vi "ACT_Loop.vi"() -> ()   [LabVIEW 2023, in "2024 AdvSwerve_ACT.lvlib"]
uses:
  2024 AdvSwerve_ACT.lvlib
  Cluster_CMD_ACT_Data.ctl
  ENUM_CMD_Mode Select.ctl
  Shared Code/TypeDefs/Cluster_CMD_Direction Data.ctl
  Shared Code/TypeDefs/Cluster_Module Velocity-Direction-Rotations.ctl
  Shared Code/TypeDefs/Level_Velocity plus-minus 1.ctl
  Shared Code/TypeDefs/Dial_Compase heading unit circle CCW positive.ctl
  Shared Code/TypeDefs/Cluster_X-Y.ctl
  Cluster_HW Output Values.ctl
  Shared Code/TypeDefs/Cluster_Swerve 4 Steer and Velocity.ctl
  Cluster_System Output Data.ctl
  Cluster_System Config_Values.ctl
  Shared Code/TypeDefs/Cluster_SW PID Config.ctl
  Shared Code/TypeDefs/Cluster_PID Gains.ctl
  Shared Code/TypeDefs/Cluster_High-Low.ctl
  Type Defs/Cluster_Length and Width.ctl
  Shared Code/TypeDefs/Cluster_Config_Swerve_Drive Param.ctl
  Shared Code/TypeDefs/Cluster_Config_Swerve_Steer Parm.ctl
  Cluster_Config Specific HW Values.ctl
  Cluster_Config Specific Data.ctl
  Shared Code/TypeDefs/ENUM_Module Position.ctl
  Cluster_Config Steer HW Values.ctl
  Shared Code/TypeDefs/Cluster_SparkMax Config_Motor Output.ctl
  <vilib>/Rock Robotics/WPI/ThirdParty/REV Robotics/REVLib/Typedef/Spark MAX Idle Mode.ctl
  Shared Code/TypeDefs/Cluster_Spark MAX Config_SLOT PID Config.ctl
  Shared Code/TypeDefs/Cluster_SparkMax Config_Smart Motion Parameters.ctl
  Cluster_Config Drive HW Values.ctl
  ENUM_ACT_State.ctl
  <vilib>/Rock Robotics/WPI/ThirdParty/Phoenix-LabVIEW/Motor Controller/Controls/CTRE_Phoenix_MotorControl_ControlMode.ctl
  <vilib>/Rock Robotics/WPI/MotorControl/WPI_MotorControlDeviceRef.ctl
  <vilib>/Rock Robotics/WPI/MotorControl/WPI_MotorControlType.ctl
  <vilib>/Rock Robotics/SystemInterfaces/DIO/FPGA_DIOPWMChannel.ctl
  <vilib>/Rock Robotics/WPI/PWM/WPI_PWMDeadband.ctl
  <vilib>/Rock Robotics/SystemInterfaces/DIO/FPGA_DIOChannel.ctl
  <vilib>/Rock Robotics/WPI/ThirdParty/Phoenix-LabVIEW/CANCoder/Controls/CTRE_Phoenix_CANcoder_DeviceRef.ctl
  ENUM_ACT_Action.ctl
  4f1f8321-3dc8-4b28-8619-20673fc77ec2.vi
  cbff3d61-3b62-444e-9844-795ae03579cd.vi
  089052c0-d540-4a78-a5cc-aeb70dbb496b.vi
  6201c2b1-dcd8-4430-86f1-9b4ee56c7753.vi
  b5508d6c-c1cc-4273-80c5-2077d34e1483.vi
  5f725c2a-0ce1-4524-8967-e83b15fdce90.vi
  bd5da564-2e8e-4505-86fc-30918feadaa2.vi
  8beda75f-c59a-4462-acc7-7c37ceab3777.vi
  47a9b741-f4a3-48b6-ae85-4ba2e502368e.vi
  e2e8a241-7810-4d95-85fd-17f3a55957a8.vi
  80d407e5-f582-430c-986f-ecd413765478.vi
  573e44c0-11f4-4bd9-ad56-904ec25dba75.vi
  e7494af9-f670-4352-9dfa-ae6ce50709ea.vi
  <vilib>/Utility/error.llb/Trim Whitespace.vi
  5f725c2a-0ce1-4524-8967-e83b15fdce90.vi/958b2683-dd4b-41b7-8ed1-41c95f63cef0.vi
  5f725c2a-0ce1-4524-8967-e83b15fdce90.vi/95f5fa9b-6175-4b34-88ee-cece92c38279.vi
  bd5da564-2e8e-4505-86fc-30918feadaa2.vi/958b2683-dd4b-41b7-8ed1-41c95f63cef0.vi
  bd5da564-2e8e-4505-86fc-30918feadaa2.vi/95f5fa9b-6175-4b34-88ee-cece92c38279.vi
  8beda75f-c59a-4462-acc7-7c37ceab3777.vi/958b2683-dd4b-41b7-8ed1-41c95f63cef0.vi
  8beda75f-c59a-4462-acc7-7c37ceab3777.vi/95f5fa9b-6175-4b34-88ee-cece92c38279.vi
  47a9b741-f4a3-48b6-ae85-4ba2e502368e.vi/958b2683-dd4b-41b7-8ed1-41c95f63cef0.vi
  47a9b741-f4a3-48b6-ae85-4ba2e502368e.vi/95f5fa9b-6175-4b34-88ee-cece92c38279.vi
  e2e8a241-7810-4d95-85fd-17f3a55957a8.vi/958b2683-dd4b-41b7-8ed1-41c95f63cef0.vi
  e2e8a241-7810-4d95-85fd-17f3a55957a8.vi/95f5fa9b-6175-4b34-88ee-cece92c38279.vi
  80d407e5-f582-430c-986f-ecd413765478.vi/958b2683-dd4b-41b7-8ed1-41c95f63cef0.vi
  80d407e5-f582-430c-986f-ecd413765478.vi/95f5fa9b-6175-4b34-88ee-cece92c38279.vi
  573e44c0-11f4-4bd9-ad56-904ec25dba75.vi/958b2683-dd4b-41b7-8ed1-41c95f63cef0.vi
  573e44c0-11f4-4bd9-ad56-904ec25dba75.vi/95f5fa9b-6175-4b34-88ee-cece92c38279.vi
  e7494af9-f670-4352-9dfa-ae6ce50709ea.vi/958b2683-dd4b-41b7-8ed1-41c95f63cef0.vi
  e7494af9-f670-4352-9dfa-ae6ce50709ea.vi/95f5fa9b-6175-4b34-88ee-cece92c38279.vi
  <vilib>/Utility/error.llb/Trim Whitespace One-Sided.vi
  5f725c2a-0ce1-4524-8967-e83b15fdce90.vi/95f5fa9b-6175-4b34-88ee-cece92c38279.vi/1c6bd52c-bbca-4d4a-a290-93ea2703fded.vi
  5f725c2a-0ce1-4524-8967-e83b15fdce90.vi/95f5fa9b-6175-4b34-88ee-cece92c38279.vi/47c2b0d5-b5fa-444e-9535-611565d375db.vi
  bd5da564-2e8e-4505-86fc-30918feadaa2.vi/95f5fa9b-6175-4b34-88ee-cece92c38279.vi/1c6bd52c-bbca-4d4a-a290-93ea2703fded.vi
  bd5da564-2e8e-4505-86fc-30918feadaa2.vi/95f5fa9b-6175-4b34-88ee-cece92c38279.vi/47c2b0d5-b5fa-444e-9535-611565d375db.vi
  8beda75f-c59a-4462-acc7-7c37ceab3777.vi/95f5fa9b-6175-4b34-88ee-cece92c38279.vi/1c6bd52c-bbca-4d4a-a290-93ea2703fded.vi
  8beda75f-c59a-4462-acc7-7c37ceab3777.vi/95f5fa9b-6175-4b34-88ee-cece92c38279.vi/47c2b0d5-b5fa-444e-9535-611565d375db.vi
  47a9b741-f4a3-48b6-ae85-4ba2e502368e.vi/95f5fa9b-6175-4b34-88ee-cece92c38279.vi/1c6bd52c-bbca-4d4a-a290-93ea2703fded.vi
  47a9b741-f4a3-48b6-ae85-4ba2e502368e.vi/95f5fa9b-6175-4b34-88ee-cece92c38279.vi/47c2b0d5-b5fa-444e-9535-611565d375db.vi
  e2e8a241-7810-4d95-85fd-17f3a55957a8.vi/95f5fa9b-6175-4b34-88ee-cece92c38279.vi/1c6bd52c-bbca-4d4a-a290-93ea2703fded.vi
  e2e8a241-7810-4d95-85fd-17f3a55957a8.vi/95f5fa9b-6175-4b34-88ee-cece92c38279.vi/47c2b0d5-b5fa-444e-9535-611565d375db.vi
  80d407e5-f582-430c-986f-ecd413765478.vi/95f5fa9b-6175-4b34-88ee-cece92c38279.vi/1c6bd52c-bbca-4d4a-a290-93ea2703fded.vi
  80d407e5-f582-430c-986f-ecd413765478.vi/95f5fa9b-6175-4b34-88ee-cece92c38279.vi/47c2b0d5-b5fa-444e-9535-611565d375db.vi
  573e44c0-11f4-4bd9-ad56-904ec25dba75.vi/95f5fa9b-6175-4b34-88ee-cece92c38279.vi/1c6bd52c-bbca-4d4a-a290-93ea2703fded.vi
  573e44c0-11f4-4bd9-ad56-904ec25dba75.vi/95f5fa9b-6175-4b34-88ee-cece92c38279.vi/47c2b0d5-b5fa-444e-9535-611565d375db.vi
  e7494af9-f670-4352-9dfa-ae6ce50709ea.vi/95f5fa9b-6175-4b34-88ee-cece92c38279.vi/1c6bd52c-bbca-4d4a-a290-93ea2703fded.vi
  e7494af9-f670-4352-9dfa-ae6ce50709ea.vi/95f5fa9b-6175-4b34-88ee-cece92c38279.vi/47c2b0d5-b5fa-444e-9535-611565d375db.vi
  RoboRIO Utilities/Global_STOP.vi
  Global_CMD_ACT_Data In.vi
  PigeonIMU/Global_SEN_Data Out.vi
  Global_ACT_Data Out.vi
  <vilib>/Utility/Data Type/Get Type Information.vi
  Shared Code/Utility/RWA/RWA/File/RWA_PC FIle Read String.vi
  Shared Code/Utility/RWA/RWA/Read Write Anything/RWA_File String.vi
  Shared Code/Utility/RWA/RWA/File/RWA_PC File Write String.vi
  <vilib>/Comparison/Equal/Equal Functor/Equal Functor.lvclass
  PigeonIMU/PigeonIMU_SEN_ts.lvlib
panel:
  in  "Set Steer Start Values":bool
  in  "Config Drive":T1={"Drive HW Ver"=0, "SparkMax Output"={"Motor Invert"=FALSE, "Ramp Rate OL (S)"=1.0, "Dead Band"=0.0, "Idle Mode"=enum."Coast"}, "Slot 0 CL"={"Gains"={"P"=0.1, "I"=0.0, "D"=0.0, "F"=0.0}, "I Zone"=0.0, "Peak Out -1 0 1"={"High"=0.0, "Low"=0.0}, "Max I Accu"=0.0}, "Slot 0 SM"={"Max Velocity"=0.0, "Max Acceleration"=0.0, "Allowed CL Error"=0.0, "Min Velocity Output"=0.0}} {"Slot 0 CL"."Gains"."F" format="%#.8f"; "Slot 0 CL"."Gains"."D" format="%#.8f"; "Slot 0 CL"."Gains"."I" format="%#.8f"; "Slot 0 CL"."Gains"."P" format="%#.8f"; "Slot 0 CL"."Peak Out -1 0 1"."Low" format="%#.8f"; "Slot 0 CL"."Peak Out -1 0 1"."High" format="%#.8f"}
  in  "Config Steer":T8={"Steer HW Ver"=0, "SparkMax Output"={"Motor Invert"=FALSE, "Ramp Rate OL (S)"=1.0, "Dead Band"=0.0, "Idle Mode"=enum."Coast"}, "Slot 0 CL"={"Gains"={"P"=1.0, "I"=0.01, "D"=0.0, "F"=0.0}, "I Zone"=10000.0, "Peak Out -1 0 1"={"High"=1.0, "Low"=-1.0}, "Max I Accu"=-1000.0}, "Slot 0 SM"={"Max Velocity"=5000.0, "Max Acceleration"=5000.0, "Allowed CL Error"=0.0, "Min Velocity Output"=0.0}} {"Slot 0 CL"."Gains"."F" format="%#.8f"; "Slot 0 CL"."Gains"."D" format="%#.8f"; "Slot 0 CL"."Gains"."I" format="%#.8f"; "Slot 0 CL"."Gains"."P" format="%#.8f"; "Slot 0 CL"."Peak Out -1 0 1"."Low" format="%#.8f"; "Slot 0 CL"."Peak Out -1 0 1"."High" format="%#.8f"}
  in  "Config Specific":T9={"Specific HW Ver"=0, "Specific Data"=[{"Motor Pos"=enum."Left-Front", "CAN Bus"="", "NEO Drive ID"=0, "NEO-Cancoder SteerID"=0, "Encoder Start Value"=0.0}, {"Motor Pos"=enum."Right-Front", "CAN Bus"="", "NEO Drive ID"=0, "NEO-Cancoder SteerID"=0, "Encoder Start Value"=0.0}, {"Motor Pos"=enum."Right-Back", "CAN Bus"="", "NEO Drive ID"=0, "NEO-Cancoder SteerID"=0, "Encoder Start Value"=0.0}, {"Motor Pos"=enum."Left-Back", "CAN Bus"="", "NEO Drive ID"=0, "NEO-Cancoder SteerID"=0, "Encoder Start Value"=0.0}]}
  in  "CMD Override":T12(tab)
  in  "Overide CMD":T13 {"Target Auto Angle" scale format="%.3f"; "Direction"."Rotate(Yaw) CCW 1 CW -1" scale=1.0..-1.0; "Direction"."Traverse"."Angle" scale format="%.3f"; "Direction"."Traverse"."Velocity" scale=-1.0..1.0 scale format="%.1f"}
  in  "Overide 1":bool caption="Overide"
  in  "Target Auto Angle":T18 scale format="%.3f"
  in  "Overide 2":bool caption="Overide"
  out "Current Time":timestamp
  in  "Config System":T20={"System Ver"=0, "Auto Angle PID"={"Gains"={"P"=0.1, "I"=0.0, "D"=0.0, "F"=0.0}, "Error Allowed"={"High"=0.0, "Low"=0.0}, "I Zone"={"High"=0.0, "Low"=0.0}, "Peak Out 0-1"={"High"=0.0, "Low"=0.0}, "Max I Accu"={"High"=0.0, "Low"=0.0}}, "Frame"={"Length"=33.0, "Width"=18.0}, "Drive Data"={"CPR"=14.0, "RevMotor/Wheel"=6.67, "Wheel Diameter (in)"=4.0}, "Speed Full Scale"=5000.0, "Steer Data"={"CPR"=1024.0}} {"Auto Angle PID"."Max I Accu"."Low" format="%#.8f"; "Auto Angle PID"."Max I Accu"."High" format="%#.8f"; "Auto Angle PID"."Gains"."F" format="%#.8f"; "Auto Angle PID"."Gains"."D" format="%#.8f"; "Auto Angle PID"."Gains"."I" format="%#.8f"; "Auto Angle PID"."Gains"."P" format="%#.8f"; "Auto Angle PID"."Error Allowed"."Low" format="%#.8f"; "Auto Angle PID"."Error Allowed"."High" format="%#.8f"; "Auto Angle PID"."I Zone"."Low" format="%#.8f"; "Auto Angle PID"."I Zone"."High" format="%#.8f"; "Auto Angle PID"."Peak Out 0-1"."Low" format="%#.8f"; "Auto Angle PID"."Peak Out 0-1"."High" format="%#.8f"}
  out "System Config":T25
  out "Sensor Read time":dbl format="%.3g"
  out "HW Output":T26 {"Swerve Read"."Back Right"."Angle" scale format="%.3f"; "Swerve Read"."Back Right"."Velocity" scale=-1.0..1.0 scale format="%.1f"; "Swerve Read"."Back Left"."Angle" scale format="%.3f"; "Swerve Read"."Back Left"."Velocity" scale=-1.0..1.0 scale format="%.1f"; "Swerve Read"."Front Left"."Angle" scale format="%.3f"; "Swerve Read"."Front Left"."Velocity" scale=-1.0..1.0 scale format="%.1f"; "Swerve Read"."Front Right"."Angle" scale format="%.3f"; "Swerve Read"."Front Right"."Velocity" scale=-1.0..1.0 scale format="%.1f"; "Pigeon Heading" scale format="%.3f"}
  in  "Read Saved Config":bool
  in  "Update Config":bool
  out "CMD":T13 {"Target Auto Angle" scale format="%.3f"; "Direction"."Rotate(Yaw) CCW 1 CW -1" scale=1.0..-1.0; "Direction"."Traverse"."Angle" scale format="%.3f"; "Direction"."Traverse"."Velocity" scale=-1.0..1.0 scale format="%.1f"}
  out "Cycle Time (S)":dbl format="%.3g"
  # "Teleop\nAuto"
  # "STOP"
  # "\"Front\" of Robot"
  # "Index 1"
  # "Index 0"
  # "Index 3"
  # "Index 2"
  # "Right Hand Rule"
  # "X"
  # "+CCW"
  # "Y"
  # "(0,0)"
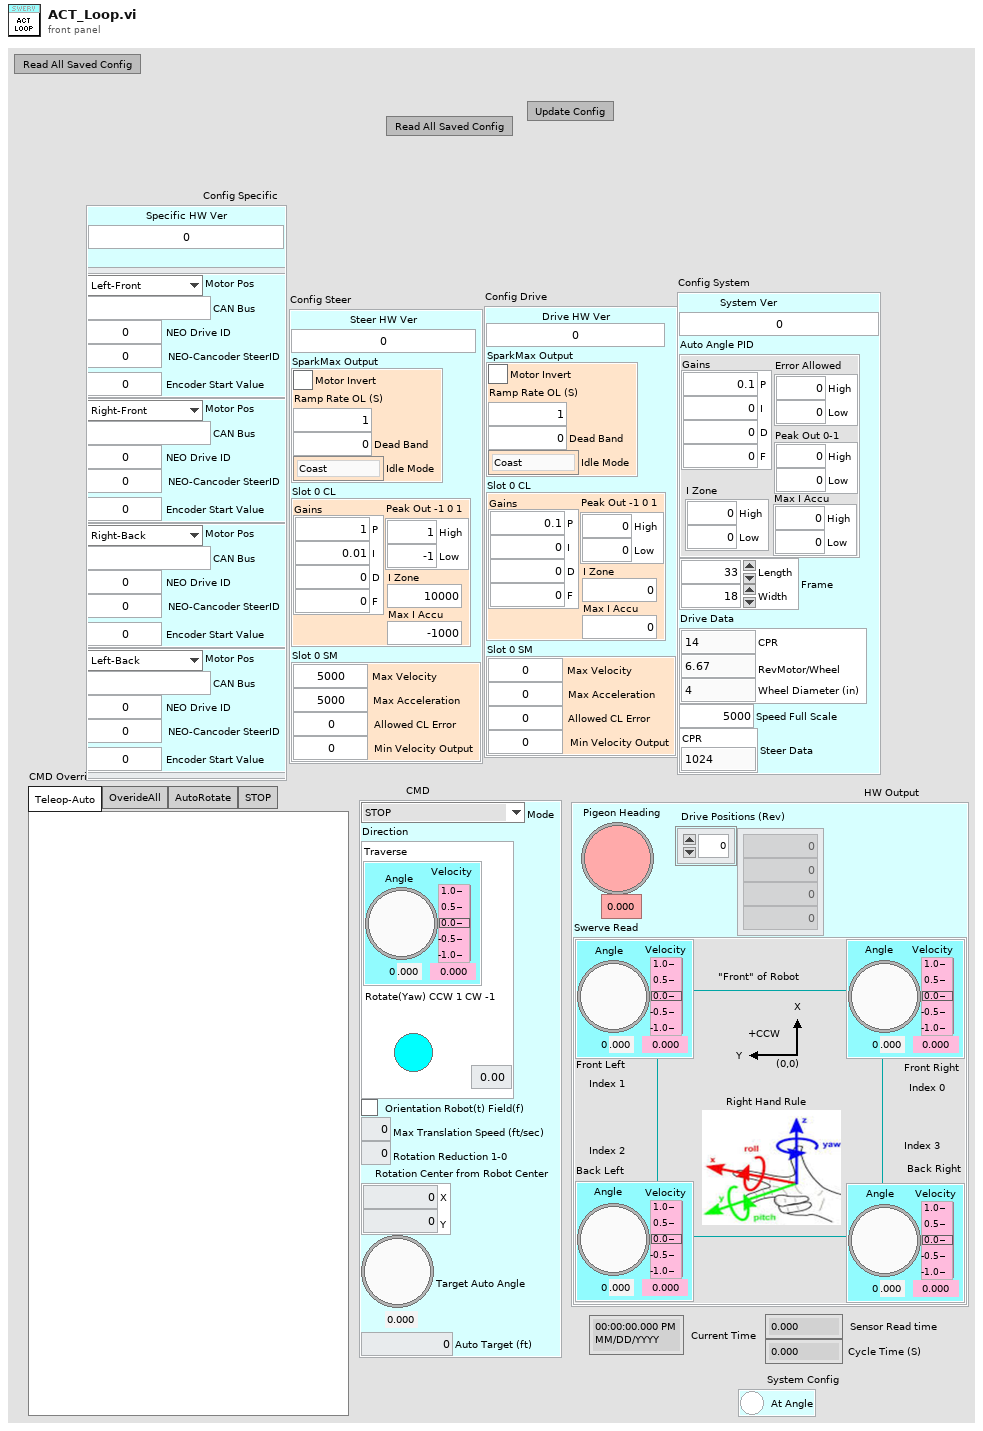
[diagram p1: front panel]
types:
  T1 = typedef "2024 AdvSwerve_ACT.lvlib/Cluster_Config Drive HW Values.ctl" = cluster{"Drive HW Ver":u64, "SparkMax Output":T2, "Slot 0 CL":T4, "Slot 0 SM":T7}
  T2 = typedef "Cluster_SparkMax Config_Motor Output.ctl" = cluster{"Motor Invert":bool, "Ramp Rate OL (S)":dbl, "Dead Band":dbl, "Idle Mode":T3}
  T3 = typedef "Spark MAX Idle Mode.ctl" = enum16{"Coast", "Brake"}
  T4 = typedef "Cluster_Spark MAX Config_SLOT PID Config.ctl" = cluster{"Gains":T5, "I Zone":dbl, "Peak Out -1 0 1":T6, "Max I Accu":dbl}
  T5 = typedef "Cluster_PID Gains.ctl" = cluster{"P":dbl, "I":dbl, "D":dbl, "F":dbl}
  T6 = typedef "Cluster_High-Low.ctl" = cluster{"High":dbl, "Low":dbl}
  T7 = typedef "Cluster_SparkMax Config_Smart Motion Parameters.ctl" = cluster{"Max Velocity":dbl, "Max Acceleration":dbl, "Allowed CL Error":dbl, "Min Velocity Output":dbl}
  T8 = typedef "2024 AdvSwerve_ACT.lvlib/Cluster_Config Steer HW Values.ctl" = cluster{"Steer HW Ver":u64, "SparkMax Output":T2, "Slot 0 CL":T4, "Slot 0 SM":T7}
  T9 = typedef "2024 AdvSwerve_ACT.lvlib/Cluster_Config Specific HW Values.ctl" = cluster{"Specific HW Ver":u64, "Specific Data":T10[]}
  T10 = typedef "2024 AdvSwerve_ACT.lvlib/Cluster_Config Specific Data.ctl" = cluster{"Motor Pos":T11, "CAN Bus":string, "NEO Drive ID":u8, "NEO-Cancoder SteerID":u8, "Encoder Start Value":dbl}
  T11 = typedef "ENUM_Module Position.ctl" = enum16{"Left-Front", "Right-Front", "Left-Back", "Right-Back"}
  T12 = enum32{"Teleop-Auto", "OverideAll", "AutoRotate", "STOP"}
  T13 = typedef "2024 AdvSwerve_ACT.lvlib/Cluster_CMD_ACT_Data.ctl" = cluster{"Mode":T14, "Direction":T15, "Orientation Robot(t) Field(f)":bool, "Max Translation Speed (ft/sec)":dbl, "Rotation Reduction 1-0":dbl, "Rotation Center from Robot Center":T19, "Target Auto Angle":T18, "Auto Target (ft)":dbl}
  T14 = typedef "2024 AdvSwerve_ACT.lvlib/ENUM_CMD_Mode Select.ctl" = enum16{"STOP", "Move", "Turret Manual", "Trans Manual Angle Auto", "Turret Auto Angle"}
  T15 = typedef "Cluster_CMD_Direction Data.ctl" = cluster{"Traverse":T16, "Rotate(Yaw) CCW 1 CW -1":dbl}
  T16 = typedef "Cluster_Module Velocity-Direction-Rotations.ctl" = cluster{"Velocity":T17, "Angle":T18, "Rotations Count":dbl}
  T17 = typedef "Level_Velocity plus-minus 1.ctl" = dbl
  T18 = typedef "Dial_Compase heading unit circle CCW positive.ctl" = dbl
  T19 = typedef "Cluster_X-Y.ctl" = cluster{"X":dbl, "Y":dbl}
  T20 = typedef "2024 AdvSwerve_ACT.lvlib/Cluster_System Config_Values.ctl" = cluster{"System Ver":u64, "Auto Angle PID":T21, "Frame":T22, "Drive Data":T23, "Speed Full Scale":dbl, "Steer Data":T24}
  T21 = typedef "Cluster_SW PID Config.ctl" = cluster{"Gains":T5, "Error Allowed":T6, "I Zone":T6, "Peak Out 0-1":T6, "Max I Accu":T6}
  T22 = typedef "Cluster_Length and Width.ctl" = cluster{"Length":dbl, "Width":dbl}
  T23 = typedef "Cluster_Config_Swerve_Drive Param.ctl" = cluster{"CPR":dbl, "RevMotor/Wheel":dbl, "Wheel Diameter (in)":dbl}
  T24 = typedef "Cluster_Config_Swerve_Steer Parm.ctl" = cluster{"CPR":dbl}
  T25 = typedef "2024 AdvSwerve_ACT.lvlib/Cluster_System Output Data.ctl" = cluster{"At Angle":bool}
  T26 = typedef "2024 AdvSwerve_ACT.lvlib/Cluster_HW Output Values.ctl" = cluster{"Pigeon Heading":T18, "Swerve Read":T27, "Drive Positions (Rev)":dbl[]}
  T27 = typedef "Cluster_Swerve 4 Steer and Velocity.ctl" = cluster{"Front Right":T16, "Front Left":T16, "Back Left":T16, "Back Right":T16}
  T28 = typedef "CTRE_Phoenix_CANcoder_DeviceRef.ctl" = cluster{"DeviceStatus":errorcluster, "Device Number":u8, "Handle":u64, "UsageFrame":u32, "Library Path":path}
  T29 = typedef "WPI_MotorControlDeviceRef.ctl" = cluster{"DeviceStatus":errorcluster, "Type":T30, "PWM":cluster{"PWM Channel":T31, "DeadBand":T32}, "CAN":cluster{"Device Number":u8, "SetOutput VI Ref":variant, "GetOutput VI Ref":variant, "Enable VI Ref":variant, "Disable VI Ref":variant, "Data":variant}, "Invert":bool, "DIO PWM":cluster{"PWM \"Enable\" Channel":T31, "DIOChannel":T33, "PWM Rate":dbl}}
  T30 = typedef "WPI_MotorControlType.ctl" = enum16{"PWM", "CAN", "DIO PWM"}
  T31 = typedef "FPGA_DIOPWMChannel.ctl" = enum8{"PWM 0", "PWM 1", "PWM 2", "PWM 3", "PWM 4", "PWM 5", "PWM 6", "PWM 7", "PWM 8", "PWM 9", "PWM MXP 0", "PWM MXP 1", "PWM MXP 2", "PWM MXP 3", "PWM MXP 4", "PWM MXP 5", "PWM MXP 6", "PWM MXP 7", "PWM MXP 8", "PWM MXP 9", "Invalid"}
  T32 = typedef "WPI_PWMDeadband.ctl" = cluster{"Name":string, "maxPositivePwm":i32, "minPositivePwm":i32, "centerPwm":i32, "maxNegativePwm":i32, "minNegativePwm":i32, "angularRange":u16}
  T33 = typedef "FPGA_DIOChannel.ctl" = enum8{"DIO 0", "DIO 1", "DIO 2", "DIO 3", "DIO 4", "DIO 5", "DIO 6", "DIO 7", "DIO 8", "DIO 9", "DIO MXP 0", "DIO MXP 1", "DIO MXP 2", "DIO MXP 3", "DIO MXP 4", "DIO MXP 5", "DIO MXP 6", "DIO MXP 7", "DIO MXP 8", "DIO MXP 9", "DIO MXP 10", "DIO MXP 11", "DIO MXP 12", "DIO MXP 13", "DIO MXP 14", "DIO MXP 15", "SPI Port CS1", "SPI Port CS2", "SPI Port CS3", "SPI Port MISO", "SPI Port MOSI", "Invalid"}
  T34 = typedef "CTRE_Phoenix_MotorControl_ControlMode.ctl" = u16
  T35 = typedef "2024 AdvSwerve_ACT.lvlib/ENUM_ACT_State.ctl" = enum16{"Startup", "Configuring", "Stopping", "Moving Mode 1", "Moving Mode 2", "Shutdown", "Initializing HW"}
  T36 = cluster{"Motor List":T11[], "Team Folder":path, "FX Ref":T29, "Steer Refs":T29[], "Drive Refs":T29[], "State":T35, "Previous State":T35, "Current Time":timestamp, "Previous Time":timestamp, "Start Time":timestamp, "Target Time (ms)":u32, "Cycle Time(S)":dbl, "Update Display":bool, "ACT Input":T13, "Config System":T20, "Max # Of Config Tries":i32, "HW Out":T26, "System Output":T25, "CAN Timeout":u32, "FX Mode":T34, "FX Set Value":dbl, "Config Specific":T9, "Swerve Set":T27, "New Cmd":bool, "Config Steer":T8, "Config Drive":T1, "HW OPEN":bool, "Steer Change":bool, "Drive Change":bool, "Specific Change":bool, "System Change":bool, "CANcoder Refs":T28[]}
  T37 = typedef "2024 AdvSwerve_ACT.lvlib/ENUM_ACT_Action.ctl" = enum16{"No Action", "Reset Time", "Reset All", "Open HW References", "Control FX Stop", "Control FX Mode 1", "Control FX Mode 2", "Set Robot Start Position", "Config HW Steer Set", "Config HW Steer Get", "Config HW Steer Save", "Config HW Steer Read", "Config HW Drive Set", "Config HW Drive Get", "Config HW Drive Save", "Config HW Drive Read", "Config HW Specific Set", "Config HW Specific Get", "Config HW Specific Save", "Config HW Specific Read", "Config System Save", "Config System Read", "Config From FP", "Start HW Steer Set", "Default HW Steer Set", "Defalut HW Drive Set"}
  T38 = cluster{"[0]":T16, "[1]":T16, "[2]":T16, "[3]":T16}
  T39 = typedef "Cluster_Unity Yaw-Pitch-Roll.ctl" = cluster{"Yaw":T18, "Pitch":T18, "Roll":T18}
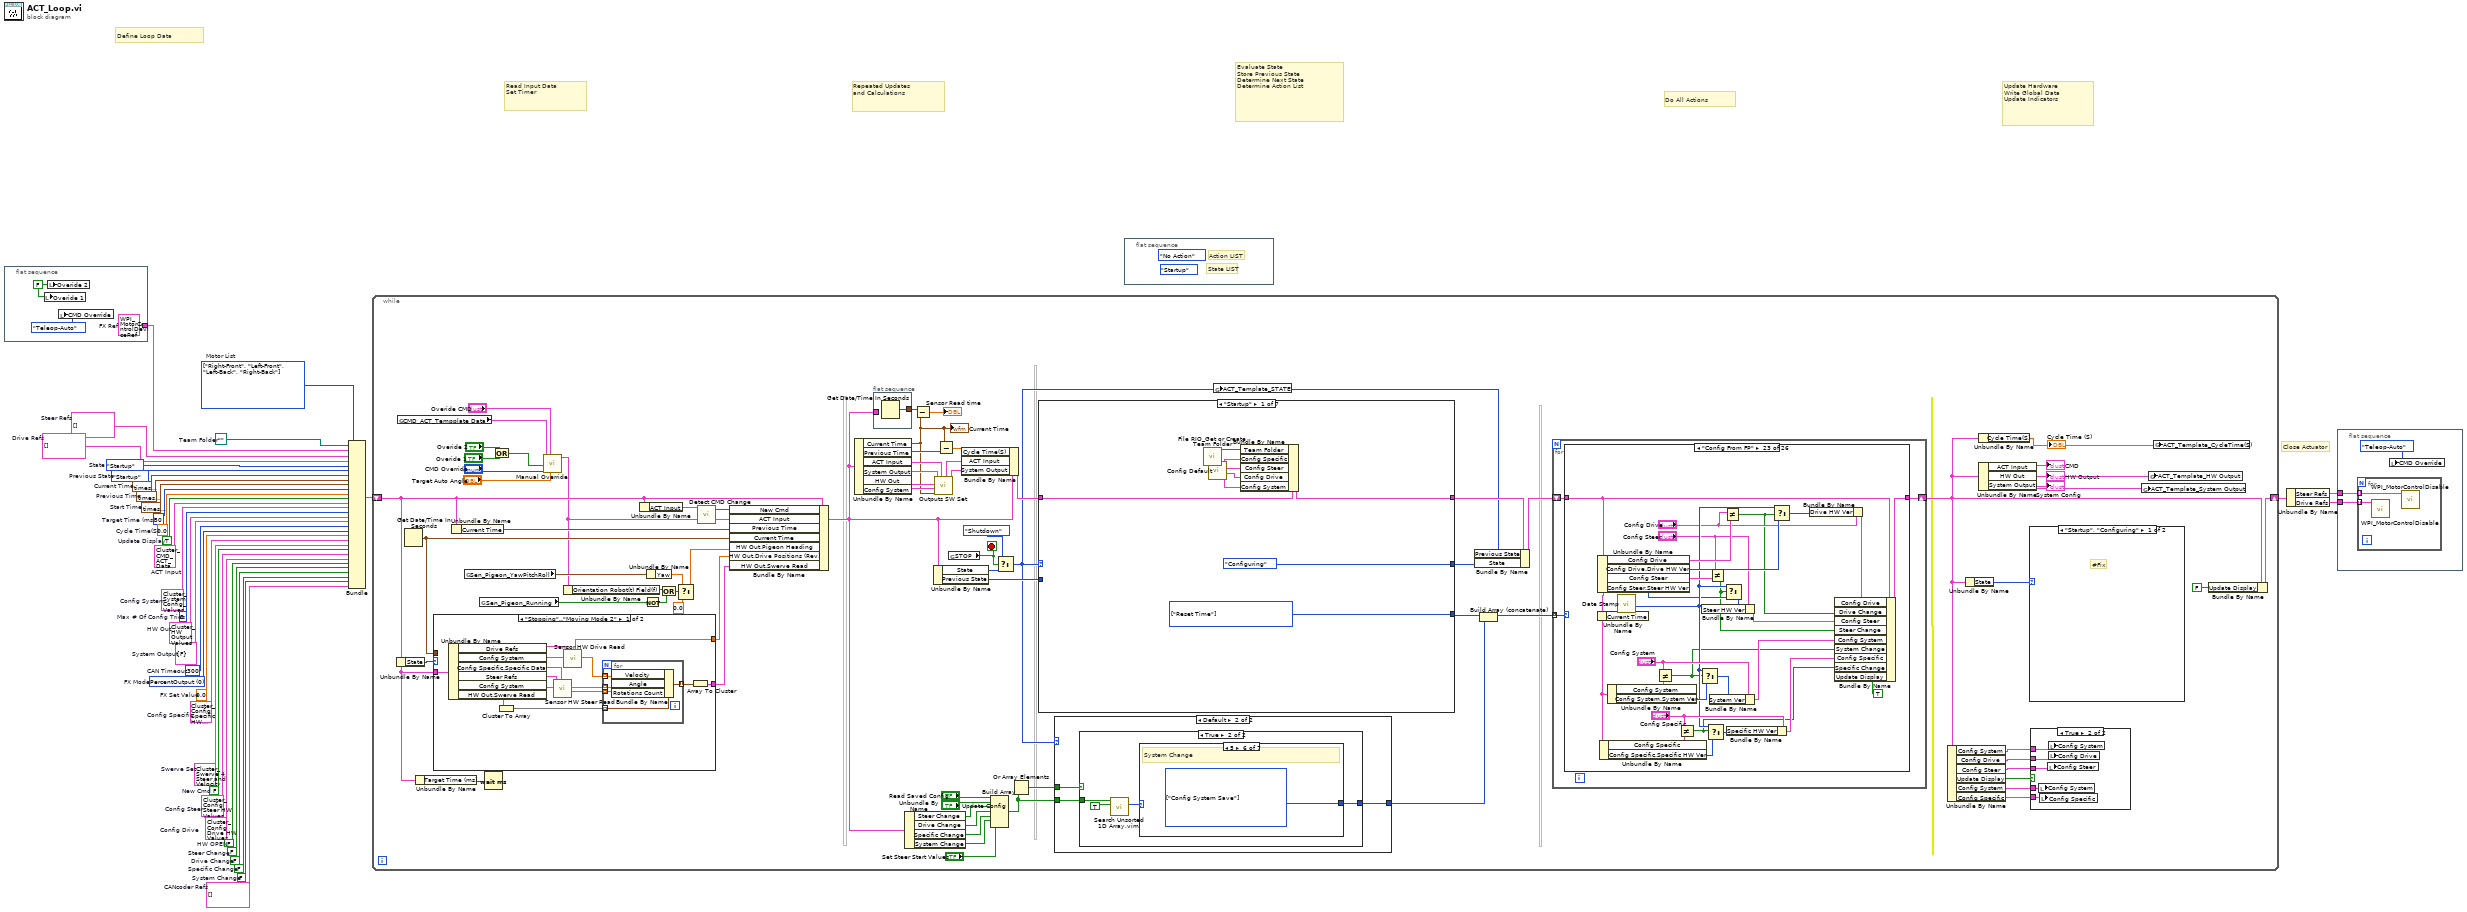
[diagram p0: block diagram]
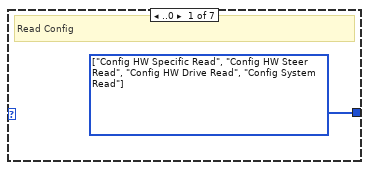
[diagram p4: hidden frame]
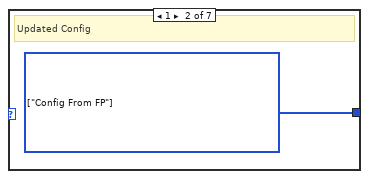
[diagram p5: hidden frame]
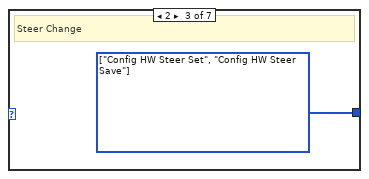
[diagram p6: hidden frame]
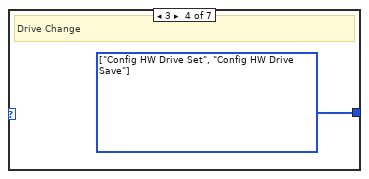
[diagram p7: hidden frame]
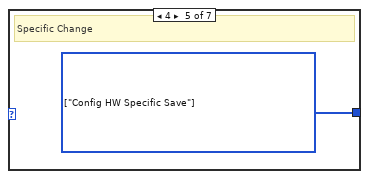
[diagram p8: hidden frame]
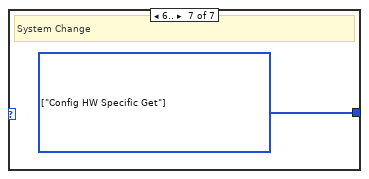
[diagram p9: hidden frame]
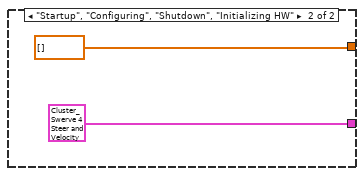
[diagram p10: hidden frame]
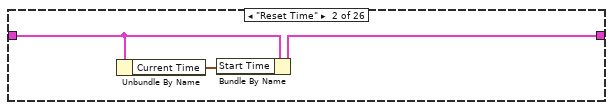
[diagram p12: hidden frame]
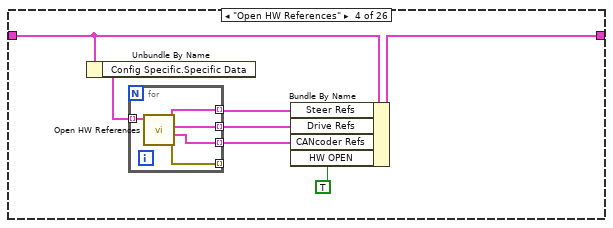
[diagram p14: hidden frame]
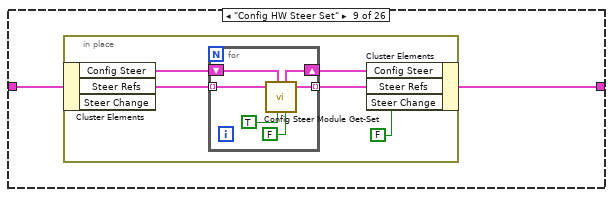
[diagram p19: hidden frame]
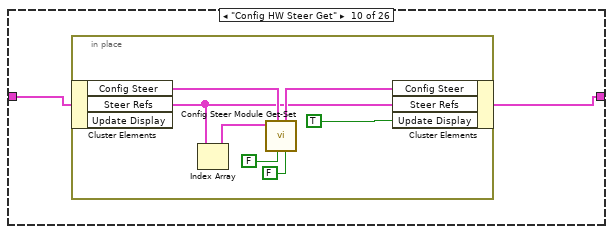
[diagram p20: hidden frame]
diagram:
  w1 = T28[] []  # CANcoder Refs
  w2 = FALSE  # System Change
  w3 = FALSE  # Specific Change
  w4 = FALSE  # Drive Change
  w5 = FALSE  # Steer Change
  w6 = FALSE  # HW OPEN
  w8 = T8 {"Steer HW Ver"=0, "SparkMax Output"={"Motor Invert"=FALSE, "Ramp Rate OL (S)"=1.0, "Dead Band"=0.0, "Idle Mode"=enum."Coast"}, "Slot 0 CL"={"Gains"={"P"=1.0, "I"=0.01, "D"=0.0, "F"=0.0}, "I Zone"=10000.0, "Peak Out -1 0 1"={"High"=1.0, "Low"=-1.0}, "Max I Accu"=-1000.0}, "Slot 0 SM"={"Max Velocity"=5000.0, "Max Acceleration"=5000.0, "Allowed CL Error"=0.0, "Min Velocity Output"=0.0}}  # Config Steer
  w7 = T1 {"Drive HW Ver"=0, "SparkMax Output"={"Motor Invert"=FALSE, "Ramp Rate OL (S)"=1.0, "Dead Band"=0.0, "Idle Mode"=enum."Coast"}, "Slot 0 CL"={"Gains"={"P"=0.1, "I"=0.0, "D"=0.0, "F"=0.0}, "I Zone"=0.0, "Peak Out -1 0 1"={"High"=0.0, "Low"=0.0}, "Max I Accu"=0.0}, "Slot 0 SM"={"Max Velocity"=0.0, "Max Acceleration"=0.0, "Allowed CL Error"=0.0, "Min Velocity Output"=0.0}}  # Config Drive
  w9 = FALSE  # New Cmd
  w10 = path ""  # Team Folder
  w12 = T27 {"Front Right"={"Velocity"=0.0, "Angle"=0.0, "Rotations Count"=0.0}, "Front Left"={"Velocity"=0.0, "Angle"=0.0, "Rotations Count"=0.0}, "Back Left"={"Velocity"=0.0, "Angle"=0.0, "Rotations Count"=0.0}, "Back Right"={"Velocity"=0.0, "Angle"=0.0, "Rotations Count"=0.0}}  # Swerve Set
  w13 = T11[] [enum."Right-Front", enum."Left-Front", enum."Left-Back", enum."Right-Back"] items=["Left-Front", "Right-Front", "Left-Back", "Right-Back"]  # Motor List
  w16 = T29[] []  # Steer Refs
  w15 = T29[] []  # Drive Refs
  w17 = T9 {"Specific HW Ver"=0, "Specific Data"=[{"Motor Pos"=enum."Left-Front", "CAN Bus"="", "NEO Drive ID"=0, "NEO-Cancoder SteerID"=0, "Encoder Start Value"=0.0}, {"Motor Pos"=enum."Right-Front", "CAN Bus"="", "NEO Drive ID"=0, "NEO-Cancoder SteerID"=0, "Encoder Start Value"=0.0}, {"Motor Pos"=enum."Right-Back", "CAN Bus"="", "NEO Drive ID"=0, "NEO-Cancoder SteerID"=0, "Encoder Start Value"=0.0}, {"Motor Pos"=enum."Left-Back", "CAN Bus"="", "NEO Drive ID"=0, "NEO-Cancoder SteerID"=0, "Encoder Start Value"=0.0}]}  # Config Specific
  w23 = T25 {"At Angle"=FALSE}  # System Output
  w25 = T20 {"System Ver"=0, "Auto Angle PID"={"Gains"={"P"=0.2, "I"=0.0, "D"=0.0, "F"=0.0}, "Error Allowed"={"High"=0.0, "Low"=0.0}, "I Zone"={"High"=0.0, "Low"=0.0}, "Peak Out 0-1"={"High"=0.0, "Low"=0.0}, "Max I Accu"={"High"=0.0, "Low"=0.0}}, "Frame"={"Length"=33.0, "Width"=18.0}, "Drive Data"={"CPR"=14.0, "RevMotor/Wheel"=6.67, "Wheel Diameter (in)"=4.0}, "Speed Full Scale"=5000.0, "Steer Data"={"CPR"=1024.0}}  # Config System
  w24 = T26 {"Pigeon Heading"=0.0, "Swerve Read"={"Front Right"={"Velocity"=0.0, "Angle"=0.0, "Rotations Count"=0.0}, "Front Left"={"Velocity"=0.0, "Angle"=0.0, "Rotations Count"=0.0}, "Back Left"={"Velocity"=0.0, "Angle"=0.0, "Rotations Count"=0.0}, "Back Right"={"Velocity"=0.0, "Angle"=0.0, "Rotations Count"=0.0}}, "Drive Positions (Rev)"=[]}  # HW Out
  w20 = 0.0  # FX Set Value
  w21 = T34 0 items=["PercentOutput"=0, "Position"=1, "Velocity"=2, "Current"=3, "Follower"=5, "MotionProfile"=6, "MotionMagic"=7, "MotionProfileArc"=10, "Disabled"=15]  # FX Mode
  w19 = u32 300  # CAN Timeout
  w18 = 3  # Max # Of Config Tries
  w27 = TRUE  # Update Display
  w30 = 0.0  # Cycle Time(S)
  w31 = ENUM_ACT_State."Startup"  # Previous State
  w32 = timestamp(0 s since 1904-01-01)  # Previous Time
  w33 = u32 50  # Target Time (ms)
  w22 = T13 {"Mode"=enum."STOP", "Direction"={"Traverse"={"Velocity"=0.0, "Angle"=0.0, "Rotations Count"=0.0}, "Rotate(Yaw) CCW 1 CW -1"=0.0}, "Orientation Robot(t) Field(f)"=FALSE, "Max Translation Speed (ft/sec)"=0.0, "Rotation Reduction 1-0"=0.0, "Rotation Center from Robot Center"={"X"=0.0, "Y"=0.0}, "Target Auto Angle"=0.0, "Auto Target (ft)"=0.0}  # ACT Input
  w34 = timestamp(0 s since 1904-01-01)  # Start Time
  w35 = timestamp(0 s since 1904-01-01)  # Current Time
  w36 = ENUM_ACT_State."Startup"  # State
  # "Close Actuator"
  # "Define Loop Data"
  # "Repeated Updates\nand Calculations"
  # "Read Input Data\nSet Timer"
  # "Evaluate State\nStore Previous State\nDetermine Next State\nDetermine Action List"
  # "Do All Actions"
  # "Update Hardware\nWrite Global Data\nUpdate Indicators"
  n1 = flat-sequence {
    tunnel: [w39] -> w28
    frame #0 {
      w37 = FALSE ("Overide 2")
      w39 = T29 {"DeviceStatus"={"status"=FALSE, "code"=0, "source"=""}, "Type"=enum."PWM", "PWM"={"PWM Channel"=enum."PWM 1", "DeadBand"={"Name"="", "maxPositivePwm"=0, "minPositivePwm"=0, "centerPwm"=0, "maxNegativePwm"=0, "minNegativePwm"=0, "angularRange"=0}}, "CAN"={"Device Number"=0, "SetOutput VI Ref"=variant(enum8{"Percent VBus", "Current", "Speed", "Position", "Voltage"} enum."Percent VBus"), "GetOutput VI Ref"=variant(refnum<k1> refnum), "Enable VI Ref"=variant(dbl 12.0), "Disable VI Ref"=variant(enum8{"Percent VBus", "Speed", "Position", "Slave", "Unchanged / Invalid", "Voltage Compensation", "Current", "Motion Profile"} enum."Percent VBus"), "Data"=variant}, "Invert"=FALSE, "DIO PWM"={"PWM \"Enable\" Channel"=enum."Invalid", "DIOChannel"=enum."Invalid", "PWM Rate"=0.0}}  # FX Ref
      n2 = local write "Overide 1"(w37) -> ()
      n3 = local write "Overide 2"(w37) -> ()
      n4 = local write "CMD Override"(T12."Teleop-Auto" ("CMD Override")) -> ()
    }
  }
  n5 = Bundle("Motor List"=w13, "Team Folder"=w10, "FX Ref"=w28, "Steer Refs"=w16, "Drive Refs"=w15, "State"=w36, "Previous State"=w31, "Current Time"=w35, "Previous Time"=w32, "Start Time"=w34, "Target Time (ms)"=w33, "Cycle Time(S)"=w30, "Update Display"=w27, "ACT Input"=w22, "Config System"=w25, "Max # Of Config Tries"=w18, "HW Out"=w24, "System Output"=w23, "CAN Timeout"=w19, "FX Mode"=w21, "FX Set Value"=w20, "Config Specific"=w17, "Swerve Set"=w12, "New Cmd"=w9, "Config Steer"=w8, "Config Drive"=w7, "HW OPEN"=w6, "Steer Change"=w5, "Drive Change"=w4, "Specific Change"=w3, "System Change"=w2, "CANcoder Refs"=w1) -> (w11:T36)  [unwired: 1 in]
  n6 = while {
    shift-right: [w97] -> w29
    shift-left: w11 -> [w60]
    stop <- w108 stop-if-true
    n7 = Unbundle By Name(w60) -> ("State"=w89:T35)
    n8 = global read "Global_CMD_ACT_Data In.vi" "CMD_ACT_Tempplate Data"() -> (w47:T13)
    n9 = Get Date/Time In Seconds() -> (seconds since 1Jan1904=w85:timestamp)
    n10 = Unbundle By Name(w60) -> ("Target Time (ms)"=w105:u32)
    n11 = case shown="\"Stopping\"..\"Moving Mode 2\"" w89 {
      tunnel: w60 -> [w138 _]
      tunnel: w85 -> [_ _]
      tunnel: [w133 T27 {"Front Right"={"Velocity"=0.0, "Angle"=0.0, "Rotations Count"=0.0}, "Front Left"={"Velocity"=0.0, "Angle"=0.0, "Rotations Count"=0.0}, "Back Left"={"Velocity"=0.0, "Angle"=0.0, "Rotations Count"=0.0}, "Back Right"={"Velocity"=0.0, "Angle"=0.0, "Rotations Count"=0.0}} ("HW Out.Swerve Read")] -> w61
      tunnel: [w128 dbl[] [] ("Drive Positions (Rev) Out")] -> w62
      frame "Stopping".."Moving Mode 2" {
        n12 = Unbundle By Name(w138) -> ("Drive Refs"=w139:T29[], "Config System"=w136:T20, "Config Specific.Specific Data"=w137:T10[], "Steer Refs"=w140:T29[], "Config System"=w127:T20, "HW Out.Swerve Read"=w135:T27)
        n13 = Cluster To Array(cluster=w135) -> (array=w134:T16[])
        n14 = call "Sensor HW Steer Read.vi"("HW Specific Config.Specific Data"=w137, "Steer"=w127, "Steer Ref"=w140) -> ("Offsets Out"=w129:dbl[], "Angles Out"=w130:dbl[])  [unwired: 5 in, 2 out]
        n15 = call "Sensor HW Drive Read.vi"("Config HW Drive Values"=w136, "Drive Ref"=w139) -> ("Drive Velocities (0-1) Out"=w131:dbl[], "Drive Positions (Rev) Out"=w128:dbl[])  [unwired: 6 in, 2 out]
        n16 = for {
          tunnel: w134 -> [w145] mode=indexing
          tunnel: [w144] -> w132 mode=indexing
          tunnel: w131 -> [w143] mode=indexing
          tunnel: w130 -> [w142] mode=indexing
          tunnel: w129 -> [w141] mode=indexing
          n17 = Bundle By Name(cluster=w145, "Velocity"=w143, "Angle"=w142, "Rotations Count"=w141) -> (w144:T16)
        }
        n18 = Array To Cluster(array=w132) -> (cluster=w133:T38)
      }
      frame "Startup", "Configuring", "Shutdown", "Initializing HW" {
      }
    }
    n19 = Unbundle By Name(w60) -> ("Current Time"=w104:timestamp)
    n20 = global read "Global_SEN_Data Out.vi" "Sen_Pigeon_YawPitchRoll"() -> (w72:T39)
    n21 = global read "Global_SEN_Data Out.vi" "Sen_Pigeon_Running"() -> (w69:bool)
    n22 = Wait (ms)(milliseconds to wait=w105) -> ()  [unwired: 1 out]
    n23 = Or(x="Overide 2", y="Overide 1") -> (x .or. y?=w44:bool)
    n24 = call "Manual Override.vi"("Target Auto Angle"="Target Auto Angle", "Overide"="Overide CMD", "CMD Override"="CMD Override", "Override"=w44, "Auto CMD"=w47) -> ("OverRide Command Out"=w58:T13)  [unwired: 6 in]
    n25 = Unbundle By Name(w58) -> ("Orientation Robot(t) Field(f)"=w73:bool)
    n26 = Unbundle By Name(w60) -> ("ACT Input"=w59:T13)
    n27 = Not(x=w69) -> (.not. x?=w68:bool)
    n28 = Unbundle By Name(w72) -> ("Yaw"=w67:T18)
    n29 = Or(x=w73, y=w68) -> (x .or. y?=w70:bool)
    n30 = Select(t=T18 0.0, s=w70, f=w67) -> (s? t:f=w66:T18)
    n31 = call "Detect CMD Change.vi"("CMD_ACT_SwerveDrive_Data"=w58, "Preious ACT Input"=w59) -> ("New Command"=w57:bool)  [unwired: 9 in]
    n32 = Bundle By Name(cluster=w60, "New Cmd"=w57, "ACT Input"=w58, "Previous Time"=w104, "Current Time"=w85, "HW Out.Pigeon Heading"=w66, "HW Out.Drive Positions (Rev)"=w62, "HW Out.Swerve Read"=w61) -> (w53:T36)
    n33 = Unbundle By Name(w53) -> ("Current Time"=w54:timestamp, "Previous Time"=w102:timestamp, "ACT Input"=w65:T13, "System Output"=w78:T25, "HW Out"=w76:T26, "Config System"=w75:T20)
    "Current Time" <- w54
    n34 = flat-sequence {
      tunnel: [w126] -> w87
      tunnel: w53 -> [_]
      frame #0 {
        n35 = Get Date/Time In Seconds() -> (seconds since 1Jan1904=w126:timestamp)
      }
    }
    n36 = Unbundle By Name(w53) -> ("Steer Change"=w52:bool, "Drive Change"=w51:bool, "Specific Change"=w50:bool, "System Change"=w49:bool)
    n37 = Subtract(x=w87, y=w54) -> (x-y=→"Sensor Read time":dbl)
    n38 = Unbundle By Name(w53) -> ("State"=w106:T35, "Previous State"=w103:T35)
    n39 = call "Outputs SW Set.vi"("Auto CMD"=w65, "Current Time"=w54, "System Config"=w75, "Sensor Values"=w76, "SW Output"=w78) -> ("SW Output Out"=w77:T25, "Auto CMD Out"=w64:T13)  [unwired: 5 in]
    n40 = Subtract(x=w54, y=w102) -> (x-y=w100:dbl)
    n41 = global read "Global_STOP.vi" "STOP"() -> (w108:bool)
    n42 = Bundle By Name(cluster=w53, "Cycle Time(S)"=w100, "ACT Input"=w64, "System Output"=w77) -> (w101:T36)
    n43 = Build Array("Read Saved Config", "Update Config", w52, w51, w50, w49, "Set Steer Start Values") -> (w81:bool[])
    n44 = Select(t=ENUM_ACT_State."Shutdown" ("State"), s=w108, f=w106) -> (s? t:f=w40:T35)
    n45 = Or Array Elements(Boolean array=w81) -> (logical OR=w82:bool)
    n46 = case shown="\"Startup\"" w40 {
      selector: w40 -> [_ _ _ _ w443 w465 _]
      tunnel: w101 -> [w346 w360 w403 w424 w444 w466 w487]
      tunnel: [w347 w360 w402 w423 w445 w467 w487] -> w110
      tunnel: [ENUM_ACT_State."Configuring" ("State") w371 w401 w422 w447 w469 ENUM_ACT_State."Shutdown" ("State")] -> w109
      tunnel: [w349 w352 w399 w420 w442 w463 w485] -> w99
      tunnel: w103 -> [_ _ _ _ _ _ _]
      frame "Startup" {
        w349 = T37[] [enum."Reset Time"] items=["No Action", "Reset Time", "Reset All", "Open HW References", "Control FX Stop", "Control FX Mode 1", "Control FX Mode 2", "Set Robot Start Position", "Config HW Steer Set", "Config HW Steer Get", "Config HW Steer Save", "Config HW Steer Read", "Config HW Drive Set", "Config HW Drive Get", "Config HW Drive Save", "Config HW Drive Read", "Config HW Specific Set", "Config HW Specific Get", "Config HW Specific Save", "Config HW Specific Read", "Config System Save", "Config System Read", "Config From FP", "Start HW Steer Set", "Default HW Steer Set", "Defalut HW Drive Set"] ("Actions")
        n47 = call "File RIO_Get or Create Team Folder.vi"() -> ("Team Files Folder"=w345:path)  [unwired: 10 in, 1 out]
        n48 = call "Config Default.vi"() -> ("System Config Out"=w341:T20, "Drive Default Out"=w342:T1, "Steer Defalut Out"=w343:T8, "Module Specific Default Out"=w344:T9)  [unwired: 8 in]
        n49 = Bundle By Name(cluster=w346, "Team Folder"=w345, "Config Specific"=w344, "Config Steer"=w343, "Config Drive"=w342, "Config System"=w341) -> (w347:T36)
      }
      frame "Configuring" {
        w355 = T37[] [enum."Open HW References"] items=["No Action", "Reset Time", "Reset All", "Open HW References", "Control FX Stop", "Control FX Mode 1", "Control FX Mode 2", "Set Robot Start Position", "Config HW Steer Set", "Config HW Steer Get", "Config HW Steer Save", "Config HW Steer Read", "Config HW Drive Set", "Config HW Drive Get", "Config HW Drive Save", "Config HW Drive Read", "Config HW Specific Set", "Config HW Specific Get", "Config HW Specific Save", "Config HW Specific Read", "Config System Save", "Config System Read", "Config From FP", "Start HW Steer Set", "Default HW Steer Set", "Defalut HW Drive Set"] ("Action")
        w354 = T37[] [] items=["No Action", "Reset Time", "Reset All", "Open HW References", "Control FX Stop", "Control FX Mode 1", "Control FX Mode 2", "Set Robot Start Position", "Config HW Steer Set", "Config HW Steer Get", "Config HW Steer Save", "Config HW Steer Read", "Config HW Drive Set", "Config HW Drive Get", "Config HW Drive Save", "Config HW Drive Read", "Config HW Specific Set", "Config HW Specific Get", "Config HW Specific Save", "Config HW Specific Read", "Config System Save", "Config System Read", "Config From FP", "Start HW Steer Set", "Default HW Steer Set", "Defalut HW Drive Set"] ("Action")
        n50 = Unbundle By Name(w360) -> ("HW OPEN"=w356:bool, "Team Folder"=w351:path)
        n51 = Unbundle By Name(w360) -> ("Config Steer"=w372:T8)
        n52 = Unbundle By Name(w360) -> ("Config Specific"=w364:T9)
        n53 = Unbundle By Name(w360) -> ("Config Drive"=w367:T1)
        n54 = Unbundle By Name(w360) -> ("Config System"=w369:T20)
        n55 = call "Config_Build Name.vim"("Config First Name"=w367) -> ("Cfg file"=w366:string)  [unwired: 9 in, 1 out]
        n56 = call "Config_Build Name.vim"("Config First Name"=w372) -> ("Cfg file"=w374:string)  [unwired: 9 in, 1 out]
        n57 = call "Config_Build Name.vim"("Config First Name"=w369) -> ("Cfg file"=w370:string)  [unwired: 9 in, 1 out]
        n58 = call "Config_Build Name.vim"("Config First Name"=w364) -> ("Cfg file"=w362:string)  [unwired: 9 in, 1 out]
        n59 = Build Path(base path=w351, name or relative path=w370) -> (appended path=w368:path)
        n60 = Build Path(base path=w351, name or relative path=w366) -> (appended path=w365:path)
        n61 = Build Path(base path=w351, name or relative path=w362) -> (appended path=w363:path)
        n62 = Build Path(base path=w351, name or relative path=w374) -> (appended path=w373:path)
        n63 = call <vilib>:"Check if File or Folder Exists.vi"("path"=w368) -> ("file or folder exists?"=w359:bool)  [unwired: 8 in, 2 out]
        n64 = call <vilib>:"Check if File or Folder Exists.vi"("path"=w365) -> ("file or folder exists?"=w357:bool)  [unwired: 8 in, 2 out]
        n65 = call <vilib>:"Check if File or Folder Exists.vi"("path"=w363) -> ("file or folder exists?"=w361:bool)  [unwired: 8 in, 2 out]
        n66 = call <vilib>:"Check if File or Folder Exists.vi"("path"=w373) -> ("file or folder exists?"=w358:bool)  [unwired: 8 in, 2 out]
        n67 = Select(t=w354, s=w356, f=w355) -> (s? t:f=w353:T37[])
        n68 = Compound Arithmetic op=AND(w361, w359, w358, w357) -> (w350:bool)
        n69 = case shown="False" w350 {
          tunnel: [ENUM_ACT_State."Configuring" ("State") ENUM_ACT_State."Stopping" ("State")] -> w371
          tunnel: [w380 w397] -> w352
          tunnel: w361 -> [w393 _]
          tunnel: w359 -> [w389 _]
          tunnel: w358 -> [w387 _]
          tunnel: w357 -> [w382 _]
          tunnel: w353 -> [w375 w396]
          frame False {
            w384 = T37[] [enum."Config HW Drive Get", enum."Config HW Drive Save"] items=["No Action", "Reset Time", "Reset All", "Open HW References", "Control FX Stop", "Control FX Mode 1", "Control FX Mode 2", "Set Robot Start Position", "Config HW Steer Set", "Config HW Steer Get", "Config HW Steer Save", "Config HW Steer Read", "Config HW Drive Set", "Config HW Drive Get", "Config HW Drive Save", "Config HW Drive Read", "Config HW Specific Set", "Config HW Specific Get", "Config HW Specific Save", "Config HW Specific Read", "Config System Save", "Config System Read", "Config From FP", "Start HW Steer Set", "Default HW Steer Set", "Defalut HW Drive Set"] ("Action")
            w383 = T37[] [] items=["No Action", "Reset Time", "Reset All", "Open HW References", "Control FX Stop", "Control FX Mode 1", "Control FX Mode 2", "Set Robot Start Position", "Config HW Steer Set", "Config HW Steer Get", "Config HW Steer Save", "Config HW Steer Read", "Config HW Drive Set", "Config HW Drive Get", "Config HW Drive Save", "Config HW Drive Read", "Config HW Specific Set", "Config HW Specific Get", "Config HW Specific Save", "Config HW Specific Read", "Config System Save", "Config System Read", "Config From FP", "Start HW Steer Set", "Default HW Steer Set", "Defalut HW Drive Set"] ("Action")
            w385 = T37[] [enum."Config HW Steer Get", enum."Config HW Steer Save"] items=["No Action", "Reset Time", "Reset All", "Open HW References", "Control FX Stop", "Control FX Mode 1", "Control FX Mode 2", "Set Robot Start Position", "Config HW Steer Set", "Config HW Steer Get", "Config HW Steer Save", "Config HW Steer Read", "Config HW Drive Set", "Config HW Drive Get", "Config HW Drive Save", "Config HW Drive Read", "Config HW Specific Set", "Config HW Specific Get", "Config HW Specific Save", "Config HW Specific Read", "Config System Save", "Config System Read", "Config From FP", "Start HW Steer Set", "Default HW Steer Set", "Defalut HW Drive Set"] ("Action")
            w386 = T37[] [] items=["No Action", "Reset Time", "Reset All", "Open HW References", "Control FX Stop", "Control FX Mode 1", "Control FX Mode 2", "Set Robot Start Position", "Config HW Steer Set", "Config HW Steer Get", "Config HW Steer Save", "Config HW Steer Read", "Config HW Drive Set", "Config HW Drive Get", "Config HW Drive Save", "Config HW Drive Read", "Config HW Specific Set", "Config HW Specific Get", "Config HW Specific Save", "Config HW Specific Read", "Config System Save", "Config System Read", "Config From FP", "Start HW Steer Set", "Default HW Steer Set", "Defalut HW Drive Set"] ("Action")
            # "Config Files Missing"
            n70 = Select(t=w386, s=w387, f=w385) -> (s? t:f=w376:T37[])
            n71 = Select(t=ENUM_ACT_Action."No Action" ("Action"), s=w389, f=ENUM_ACT_Action."Config System Save" ("Action")) -> (s? t:f=w378:T37)
            n72 = Select(t=ENUM_ACT_Action."No Action" ("Action"), s=w393, f=ENUM_ACT_Action."Config HW Specific Save" ("Action")) -> (s? t:f=w377:T37)
            n73 = Select(t=w383, s=w382, f=w384) -> (s? t:f=w379:T37[])
            n74 = Build Array (concatenate)(w377, w378, w375, w376, w379) -> (w380:T37[])
          }
          frame True {
            w395 = T37[] [enum."Config HW Specific Read", enum."Config System Read", enum."Config HW Drive Read", enum."Config HW Steer Read"] items=["No Action", "Reset Time", "Reset All", "Open HW References", "Control FX Stop", "Control FX Mode 1", "Control FX Mode 2", "Set Robot Start Position", "Config HW Steer Set", "Config HW Steer Get", "Config HW Steer Save", "Config HW Steer Read", "Config HW Drive Set", "Config HW Drive Get", "Config HW Drive Save", "Config HW Drive Read", "Config HW Specific Set", "Config HW Specific Get", "Config HW Specific Save", "Config HW Specific Read", "Config System Save", "Config System Read", "Config From FP", "Start HW Steer Set", "Default HW Steer Set", "Defalut HW Drive Set"] ("Actions")
            w394 = T37[] [enum."Default HW Steer Set", enum."Defalut HW Drive Set", enum."Config HW Steer Set", enum."Config HW Specific Set", enum."Config HW Drive Set", enum."Start HW Steer Set"] items=["No Action", "Reset Time", "Reset All", "Open HW References", "Control FX Stop", "Control FX Mode 1", "Control FX Mode 2", "Set Robot Start Position", "Config HW Steer Set", "Config HW Steer Get", "Config HW Steer Save", "Config HW Steer Read", "Config HW Drive Set", "Config HW Drive Get", "Config HW Drive Save", "Config HW Drive Read", "Config HW Specific Set", "Config HW Specific Get", "Config HW Specific Save", "Config HW Specific Read", "Config System Save", "Config System Read", "Config From FP", "Start HW Steer Set", "Default HW Steer Set", "Defalut HW Drive Set"] ("Actions")
            # "All Config File are present"
            n75 = Build Array (concatenate)(w395, w396, w394) -> (w397:T37[])
          }
        }
      }
      frame "Stopping" {
        (unwired) TRUE
        w400 = T37[] [enum."Control FX Stop"] items=["No Action", "Reset Time", "Reset All", "Open HW References", "Control FX Stop", "Control FX Mode 1", "Control FX Mode 2", "Set Robot Start Position", "Config HW Steer Set", "Config HW Steer Get", "Config HW Steer Save", "Config HW Steer Read", "Config HW Drive Set", "Config HW Drive Get", "Config HW Drive Save", "Config HW Drive Read", "Config HW Specific Set", "Config HW Specific Get", "Config HW Specific Save", "Config HW Specific Read", "Config System Save", "Config System Read", "Config From FP", "Start HW Steer Set", "Default HW Steer Set", "Defalut HW Drive Set"] ("Actions")
        n76 = Unbundle By Name(w403) -> ("ACT Input.Mode"=w404:T14)
        n77 = case shown="\"STOP\"" w404 {
          tunnel: w403 -> [w407 w410 w413 w416 w419]
          tunnel: [w407 w410 w413 w416 w419] -> w402
          tunnel: [ENUM_ACT_State."Stopping" ("State") ENUM_ACT_State."Moving Mode 1" ("State") ENUM_ACT_State."Moving Mode 2" ("State") ENUM_ACT_State."Moving Mode 2" ("State") ENUM_ACT_State."Moving Mode 2" ("State")] -> w401
          tunnel: [w405 w408 w411 w414 w417] -> w399
          tunnel: w400 -> [w405 w408 w411 w414 w417]
          frame "STOP" {
          }
          frame "Move" {
          }
          frame "Turret Manual" {
          }
          frame "Trans Manual Angle Auto" {
          }
          frame "Turret Auto Angle" {
          }
        }
      }
      frame "Initializing HW" {
        (unwired) TRUE
        w421 = T37[] [enum."Control FX Stop"] items=["No Action", "Reset Time", "Reset All", "Open HW References", "Control FX Stop", "Control FX Mode 1", "Control FX Mode 2", "Set Robot Start Position", "Config HW Steer Set", "Config HW Steer Get", "Config HW Steer Save", "Config HW Steer Read", "Config HW Drive Set", "Config HW Drive Get", "Config HW Drive Save", "Config HW Drive Read", "Config HW Specific Set", "Config HW Specific Get", "Config HW Specific Save", "Config HW Specific Read", "Config System Save", "Config System Read", "Config From FP", "Start HW Steer Set", "Default HW Steer Set", "Defalut HW Drive Set"] ("Actions")
        n78 = Unbundle By Name(w424) -> ("ACT Input.Mode"=w425:T14)
        n79 = case shown="\"Trans Manual Angle Auto\"" w425 {
          tunnel: w424 -> [w428 w431 w434 w437 w440]
          tunnel: [w428 w431 w434 w437 w440] -> w423
          tunnel: [ENUM_ACT_State."Stopping" ("State") ENUM_ACT_State."Moving Mode 1" ("State") ENUM_ACT_State."Moving Mode 2" ("State") ENUM_ACT_State."Moving Mode 2" ("State") ENUM_ACT_State."Moving Mode 2" ("State")] -> w422
          tunnel: [w426 w429 w432 w435 w438] -> w420
          tunnel: w421 -> [w426 w429 w432 w435 w438]
          frame "STOP" {
          }
          frame "Move" {
          }
          frame "Turret Manual" {
          }
          frame "Trans Manual Angle Auto" {
          }
          frame "Turret Auto Angle" {
          }
        }
      }
      frame "Moving Mode 1" {
        w441 = T37[] [enum."Control FX Stop"] items=["No Action", "Reset Time", "Reset All", "Open HW References", "Control FX Stop", "Control FX Mode 1", "Control FX Mode 2", "Set Robot Start Position", "Config HW Steer Set", "Config HW Steer Get", "Config HW Steer Save", "Config HW Steer Read", "Config HW Drive Set", "Config HW Drive Get", "Config HW Drive Save", "Config HW Drive Read", "Config HW Specific Set", "Config HW Specific Get", "Config HW Specific Save", "Config HW Specific Read", "Config System Save", "Config System Read", "Config From FP", "Start HW Steer Set", "Default HW Steer Set", "Defalut HW Drive Set"] ("Actions")
        n80 = Unbundle By Name(w444) -> ("ACT Input.Mode"=w446:T14)
        n81 = case shown="\"Turret Auto Angle\"" w446 {
          tunnel: [ENUM_ACT_State."Stopping" ("State") ENUM_ACT_State."Moving Mode 2" ("State") ENUM_ACT_State."Moving Mode 2" ("State") ENUM_ACT_State."Moving Mode 2" ("State") w461] -> w447
          tunnel: w444 -> [w450 w453 w456 w459 w462]
          tunnel: [w450 w453 w456 w459 w462] -> w445
          tunnel: w443 -> [_ _ _ _ w461]
          tunnel: [w448 w451 w454 w457 w460] -> w442
          tunnel: w441 -> [w448 w451 w454 w457 _]
          frame "STOP" {
          }
          frame "Turret Manual" {
          }
          frame "Trans Manual Angle Auto" {
          }
          frame "Turret Auto Angle" {
          }
          frame "Move" {
            w460 = T37[] [enum."Control FX Mode 1"] items=["No Action", "Reset Time", "Reset All", "Open HW References", "Control FX Stop", "Control FX Mode 1", "Control FX Mode 2", "Set Robot Start Position", "Config HW Steer Set", "Config HW Steer Get", "Config HW Steer Save", "Config HW Steer Read", "Config HW Drive Set", "Config HW Drive Get", "Config HW Drive Save", "Config HW Drive Read", "Config HW Specific Set", "Config HW Specific Get", "Config HW Specific Save", "Config HW Specific Read", "Config System Save", "Config System Read", "Config From FP", "Start HW Steer Set", "Default HW Steer Set", "Defalut HW Drive Set"] ("Actions")
          }
        }
      }
      frame "Moving Mode 2" {
        w464 = T37[] [enum."Control FX Stop"] items=["No Action", "Reset Time", "Reset All", "Open HW References", "Control FX Stop", "Control FX Mode 1", "Control FX Mode 2", "Set Robot Start Position", "Config HW Steer Set", "Config HW Steer Get", "Config HW Steer Save", "Config HW Steer Read", "Config HW Drive Set", "Config HW Drive Get", "Config HW Drive Save", "Config HW Drive Read", "Config HW Specific Set", "Config HW Specific Get", "Config HW Specific Save", "Config HW Specific Read", "Config System Save", "Config System Read", "Config From FP", "Start HW Steer Set", "Default HW Steer Set", "Defalut HW Drive Set"] ("Actions")
        n82 = Unbundle By Name(w466) -> ("ACT Input.Mode"=w468:T14)
        n83 = case shown="\"Turret Auto Angle\"" w468 {
          tunnel: [ENUM_ACT_State."Stopping" ("State") w473 w476 w479 ENUM_ACT_State."Moving Mode 1" ("State")] -> w469
          tunnel: w466 -> [w472 w475 w478 w481 w484]
          tunnel: [w472 w475 w478 w481 w484] -> w467
          tunnel: w465 -> [_ w473 w476 w479 _]
          tunnel: [w470 w474 w477 w480 w482] -> w463
          tunnel: w464 -> [w470 _ _ _ w482]
          frame "STOP" {
          }
          frame "Turret Manual" {
            w474 = T37[] [enum."Control FX Mode 2"] items=["No Action", "Reset Time", "Reset All", "Open HW References", "Control FX Stop", "Control FX Mode 1", "Control FX Mode 2", "Set Robot Start Position", "Config HW Steer Set", "Config HW Steer Get", "Config HW Steer Save", "Config HW Steer Read", "Config HW Drive Set", "Config HW Drive Get", "Config HW Drive Save", "Config HW Drive Read", "Config HW Specific Set", "Config HW Specific Get", "Config HW Specific Save", "Config HW Specific Read", "Config System Save", "Config System Read", "Config From FP", "Start HW Steer Set", "Default HW Steer Set", "Defalut HW Drive Set"] ("Actions")
          }
          frame "Trans Manual Angle Auto" {
            w477 = T37[] [enum."Control FX Mode 2"] items=["No Action", "Reset Time", "Reset All", "Open HW References", "Control FX Stop", "Control FX Mode 1", "Control FX Mode 2", "Set Robot Start Position", "Config HW Steer Set", "Config HW Steer Get", "Config HW Steer Save", "Config HW Steer Read", "Config HW Drive Set", "Config HW Drive Get", "Config HW Drive Save", "Config HW Drive Read", "Config HW Specific Set", "Config HW Specific Get", "Config HW Specific Save", "Config HW Specific Read", "Config System Save", "Config System Read", "Config From FP", "Start HW Steer Set", "Default HW Steer Set", "Defalut HW Drive Set"] ("Actions")
          }
          frame "Turret Auto Angle" {
            w480 = T37[] [enum."Control FX Mode 2"] items=["No Action", "Reset Time", "Reset All", "Open HW References", "Control FX Stop", "Control FX Mode 1", "Control FX Mode 2", "Set Robot Start Position", "Config HW Steer Set", "Config HW Steer Get", "Config HW Steer Save", "Config HW Steer Read", "Config HW Drive Set", "Config HW Drive Get", "Config HW Drive Save", "Config HW Drive Read", "Config HW Specific Set", "Config HW Specific Get", "Config HW Specific Save", "Config HW Specific Read", "Config System Save", "Config System Read", "Config From FP", "Start HW Steer Set", "Default HW Steer Set", "Defalut HW Drive Set"] ("Actions")
          }
          frame "Move" {
          }
        }
      }
      frame "Shutdown" {
        w485 = T37[] [enum."Reset All"] items=["No Action", "Reset Time", "Reset All", "Open HW References", "Control FX Stop", "Control FX Mode 1", "Control FX Mode 2", "Set Robot Start Position", "Config HW Steer Set", "Config HW Steer Get", "Config HW Steer Save", "Config HW Steer Read", "Config HW Drive Set", "Config HW Drive Get", "Config HW Drive Save", "Config HW Drive Read", "Config HW Specific Set", "Config HW Specific Get", "Config HW Specific Save", "Config HW Specific Read", "Config System Save", "Config System Read", "Config From FP", "Start HW Steer Set", "Default HW Steer Set", "Defalut HW Drive Set"] ("Actions")
      }
    }
    n84 = case shown="Default" w40 {
      tunnel: w82 -> [_ w114]
      tunnel: w81 -> [_ w113]
      tunnel: [_ w112] -> w80
      frame "Startup", "Configuring", "Shutdown" {
      }
      frame Default {
        n85 = case shown="True" w114 {
          tunnel: w113 -> [_ w117]
          tunnel: [_ w115] -> w112
          frame False {
          }
          frame True {
            n86 = call "Search Unsorted 1D Array.vim"("element"=TRUE, "unsorted 1D array"=w117) -> ("index of element"=w116:i32)  [unwired: 9 in]
            n87 = case shown="5" w116 {
              tunnel: [w119 w120 w121 w122 w123 w124 w125] -> w115
              frame ..0 {
                w119 = T37[] [enum."Config HW Specific Read", enum."Config HW Steer Read", enum."Config HW Drive Read", enum."Config System Read"] items=["No Action", "Reset Time", "Reset All", "Open HW References", "Control FX Stop", "Control FX Mode 1", "Control FX Mode 2", "Set Robot Start Position", "Config HW Steer Set", "Config HW Steer Get", "Config HW Steer Save", "Config HW Steer Read", "Config HW Drive Set", "Config HW Drive Get", "Config HW Drive Save", "Config HW Drive Read", "Config HW Specific Set", "Config HW Specific Get", "Config HW Specific Save", "Config HW Specific Read", "Config System Save", "Config System Read", "Config From FP", "Start HW Steer Set", "Default HW Steer Set", "Defalut HW Drive Set"] ("Actions")
                # "Read Config"
              }
              frame 1 {
                w120 = T37[] [enum."Config From FP"] items=["No Action", "Reset Time", "Reset All", "Open HW References", "Control FX Stop", "Control FX Mode 1", "Control FX Mode 2", "Set Robot Start Position", "Config HW Steer Set", "Config HW Steer Get", "Config HW Steer Save", "Config HW Steer Read", "Config HW Drive Set", "Config HW Drive Get", "Config HW Drive Save", "Config HW Drive Read", "Config HW Specific Set", "Config HW Specific Get", "Config HW Specific Save", "Config HW Specific Read", "Config System Save", "Config System Read", "Config From FP", "Start HW Steer Set", "Default HW Steer Set", "Defalut HW Drive Set"] ("Actions")
                # "Updated Config"
              }
              frame 2 {
                w121 = T37[] [enum."Config HW Steer Set", enum."Config HW Steer Save"] items=["No Action", "Reset Time", "Reset All", "Open HW References", "Control FX Stop", "Control FX Mode 1", "Control FX Mode 2", "Set Robot Start Position", "Config HW Steer Set", "Config HW Steer Get", "Config HW Steer Save", "Config HW Steer Read", "Config HW Drive Set", "Config HW Drive Get", "Config HW Drive Save", "Config HW Drive Read", "Config HW Specific Set", "Config HW Specific Get", "Config HW Specific Save", "Config HW Specific Read", "Config System Save", "Config System Read", "Config From FP", "Start HW Steer Set", "Default HW Steer Set", "Defalut HW Drive Set"] ("Actions")
                # "Steer Change"
              }
              frame 3 {
                w122 = T37[] [enum."Config HW Drive Set", enum."Config HW Drive Save"] items=["No Action", "Reset Time", "Reset All", "Open HW References", "Control FX Stop", "Control FX Mode 1", "Control FX Mode 2", "Set Robot Start Position", "Config HW Steer Set", "Config HW Steer Get", "Config HW Steer Save", "Config HW Steer Read", "Config HW Drive Set", "Config HW Drive Get", "Config HW Drive Save", "Config HW Drive Read", "Config HW Specific Set", "Config HW Specific Get", "Config HW Specific Save", "Config HW Specific Read", "Config System Save", "Config System Read", "Config From FP", "Start HW Steer Set", "Default HW Steer Set", "Defalut HW Drive Set"] ("Actions")
                # "Drive Change"
              }
              frame 4 {
                w123 = T37[] [enum."Config HW Specific Save"] items=["No Action", "Reset Time", "Reset All", "Open HW References", "Control FX Stop", "Control FX Mode 1", "Control FX Mode 2", "Set Robot Start Position", "Config HW Steer Set", "Config HW Steer Get", "Config HW Steer Save", "Config HW Steer Read", "Config HW Drive Set", "Config HW Drive Get", "Config HW Drive Save", "Config HW Drive Read", "Config HW Specific Set", "Config HW Specific Get", "Config HW Specific Save", "Config HW Specific Read", "Config System Save", "Config System Read", "Config From FP", "Start HW Steer Set", "Default HW Steer Set", "Defalut HW Drive Set"] ("Actions")
                # "Specific Change"
              }
              frame 5 {
                w124 = T37[] [enum."Config System Save"] items=["No Action", "Reset Time", "Reset All", "Open HW References", "Control FX Stop", "Control FX Mode 1", "Control FX Mode 2", "Set Robot Start Position", "Config HW Steer Set", "Config HW Steer Get", "Config HW Steer Save", "Config HW Steer Read", "Config HW Drive Set", "Config HW Drive Get", "Config HW Drive Save", "Config HW Drive Read", "Config HW Specific Set", "Config HW Specific Get", "Config HW Specific Save", "Config HW Specific Read", "Config System Save", "Config System Read", "Config From FP", "Start HW Steer Set", "Default HW Steer Set", "Defalut HW Drive Set"] ("Actions")
                # "System Change"
              }
              frame 6.. {
                w125 = T37[] [enum."Config HW Specific Get"] items=["No Action", "Reset Time", "Reset All", "Open HW References", "Control FX Stop", "Control FX Mode 1", "Control FX Mode 2", "Set Robot Start Position", "Config HW Steer Set", "Config HW Steer Get", "Config HW Steer Save", "Config HW Steer Read", "Config HW Drive Set", "Config HW Drive Get", "Config HW Drive Save", "Config HW Drive Read", "Config HW Specific Set", "Config HW Specific Get", "Config HW Specific Save", "Config HW Specific Read", "Config System Save", "Config System Read", "Config From FP", "Start HW Steer Set", "Default HW Steer Set", "Defalut HW Drive Set"] ("Actions")
                # "System Change"
              }
            }
          }
        }
      }
    }
    n88 = global write "Global_ACT_Data Out.vi" "ACT_Template_STATE"(w40) -> ()
    n89 = Bundle By Name(cluster=w110, "Previous State"=w40, "State"=w109) -> (w111:T36)
    n90 = Build Array (concatenate)(w99, w80) -> (w95:T37[])
    n91 = for {
      tunnel: w95 -> [w150] mode=indexing
      shift-right: [w149] -> w94
      shift-left: w111 -> [w148]
      n92 = case shown="\"Config From FP\"" w150 {
        tunnel: w148 -> [w151 w154 w155 w161 w168 w169 w170 w171 w173 w186 w199 w207 w210 w223 w237 w245 w251 w262 w274 w281 w288 w295 w308 w326 w328 w335]
        tunnel: [w151 w153 w155 w162 w168 w169 w170 w171 w172 w185 w200 w208 w209 w222 w238 w246 w253 w264 w275 w282 w289 w296 w309 w326 w327 w334] -> w149
        frame "No Action" {
        }
        frame "Reset Time" {
          n93 = Unbundle By Name(w154) -> ("Current Time"=w152:timestamp)
          n94 = Bundle By Name(cluster=w154, "Start Time"=w152) -> (w153:T36)
        }
        frame "Reset All" {
        }
        frame "Open HW References" {
          n95 = Unbundle By Name(w161) -> ("Config Specific.Specific Data"=w160:T10[])
          n96 = for {
            tunnel: w160 -> [w167] mode=indexing
            tunnel: [w165] -> w159 mode=indexing
            tunnel: [w166] -> w158 mode=indexing
            tunnel: [w164] -> w156 mode=indexing
            tunnel: [w163] -> _ mode=indexing
            n97 = call "Open HW References.vi"("Module Azimuth Config Data"=w167) -> ("Error Out"=w163:errorcluster, "CANcoder Ref Out"=w164:T28, "Module Drive Ref Out"=w166:T29, "Module Steer Ref Out"=w165:T29)  [unwired: 7 in]
          }
          n98 = Bundle By Name(cluster=w161, "Steer Refs"=w159, "Drive Refs"=w158, "CANcoder Refs"=w156, "HW OPEN"=TRUE) -> (w162:T36)
        }
        frame "Control FX Stop" {
          # "#Fix"
        }
        frame "Control FX Mode 1" {
          # "#Fix"
        }
        frame "Control FX Mode 2" {
          # "#Fix"
        }
        frame "Set Robot Start Position" {
          # "#Fix"
        }
        frame "Config HW Steer Set" {
          n99 = in-place {
            n100 = in-place-cluster #1(w173) -> ("Config Steer"=w176:T8, "Steer Refs"=w178:T29[])  [unwired: 1 out]
            n101 = for {
              tunnel: w178 -> [w184] mode=indexing
              tunnel: [w183] -> w177 mode=indexing
              shift-right: [w181] -> w175
              shift-left: w176 -> [w182]
              n102 = call "Config Steer Module Get-Set.vi"("Start With Default"=FALSE, "Get(f) Set(t)"=TRUE, "Set Steer Values"=w182, "Steer Refs"=w184) -> ("Steer Refs Out"=w183:T29, "Steer Config Out"=w181:T8)  [unwired: 5 in, 1 out]
            }
            n103 = in-place-cluster #1("Config Steer"=w175, "Steer Refs"=w177, "Steer Change"=FALSE ("Update Display")) -> (w172:T36)
          }
        }
        frame "Config HW Steer Get" {
          n104 = in-place {
            n105 = in-place-cluster #2(w186) -> ("Config Steer"=w193:T8, "Steer Refs"=w188:T29[])  [unwired: 1 out]
            n106 = Index Array(array=w188) -> (element=w189:T29)  [unwired: 1 in]
            n107 = call "Config Steer Module Get-Set.vi"("Start With Default"=FALSE, "Get(f) Set(t)"=FALSE, "Set Steer Values"=w193, "Steer Refs"=w189) -> ("Steer Config Out"=w192:T8)  [unwired: 5 in, 2 out]
            n108 = in-place-cluster #2("Config Steer"=w192, "Steer Refs"=w188, "Update Display"=TRUE) -> (w185:T36)
          }
        }
        frame "Config HW Steer Save" {
          n109 = Unbundle By Name(w199) -> ("Team Folder"=w196:path, "Config Steer"=w198:T8)
          n110 = call "RWA_File Config.vim"("Read(f) Save(t)"=TRUE ("Read(f) Write(t)"), "Target Folder Folder"=w196, "Any Config"=w198) -> ("Any Config Out"=w197:T8)  [unwired: 4 in, 4 out]
          n111 = Bundle By Name(cluster=w199, "Config Steer"=w197, "Steer Change"=FALSE) -> (w200:T36)
        }
        frame "Config HW Steer Read" {
          n112 = Unbundle By Name(w207) -> ("Team Folder"=w206:path, "Config Steer"=w202:T8)
          n113 = call "RWA_File Config.vim"("Read(f) Save(t)"=FALSE ("Read(f) Write(t)"), "Target Folder Folder"=w206, "Any Config"=w202) -> ("Any Config Out"=w203:T8)  [unwired: 4 in, 4 out]
          n114 = Not Equal?(x=w202, y=w203) -> (x != y?=w201:bool)
          n115 = Bundle By Name(cluster=w207, "Steer Change"=w201, "Config Steer"=w203, "Update Display"=TRUE) -> (w208:T36)
        }
        frame "Config HW Drive Set" {
          n116 = in-place {
            n117 = in-place-cluster #3(w210) -> ("Config Drive"=w213:T1, "Drive Refs"=w215:T29[])  [unwired: 1 out]
            n118 = for {
              tunnel: w215 -> [w221] mode=indexing
              tunnel: [w220] -> w214 mode=indexing
              shift-right: [w218] -> w212
              shift-left: w213 -> [w219]
              n119 = call "Config Drive Module Get-Set.vi"("Start with Default"=FALSE ("Start With Default"), "Get(f) Set(t)"=TRUE, "Set Drive Config"=w219, "Drive Refs"=w221) -> ("Drive Refs Out"=w220:T29, "Drive Config Out"=w218:T1)  [unwired: 5 in, 1 out]
            }
            n120 = in-place-cluster #3("Config Drive"=w212, "Drive Refs"=w214, "Drive Change"=FALSE) -> (w209:T36)
          }
        }
        frame "Config HW Drive Get" {
          n121 = in-place {
            n122 = in-place-cluster #4(w223) -> ("Config Drive"=w231:T1, "Drive Refs"=w226:T29[])  [unwired: 1 out]
            n123 = Index Array(array=w226, index=3) -> (element=w227:T29)
            n124 = call "Config Drive Module Get-Set.vi"("Start with Default"=FALSE ("Start With Default"), "Get(f) Set(t)"=FALSE, "Set Drive Config"=w231, "Drive Refs"=w227) -> ("Drive Config Out"=w230:T1)  [unwired: 5 in, 2 out]
            n125 = in-place-cluster #4("Config Drive"=w230, "Drive Refs"=w226, "Update Display"=TRUE) -> (w222:T36)
          }
        }
        frame "Config HW Drive Save" {
          n126 = Unbundle By Name(w237) -> ("Team Folder"=w234:path, "Config Drive"=w236:T1)
          n127 = call "RWA_File Config.vim"("Read(f) Save(t)"=TRUE ("Read(f) Write(t)"), "Target Folder Folder"=w234, "Any Config"=w236) -> ("Any Config Out"=w235:T1)  [unwired: 4 in, 4 out]
          n128 = Bundle By Name(cluster=w237, "Config Drive"=w235, "Drive Change"=FALSE) -> (w238:T36)
        }
        frame "Config HW Drive Read" {
          n129 = Unbundle By Name(w245) -> ("Team Folder"=w244:path, "Config Drive"=w240:T1)
          n130 = call "RWA_File Config.vim"("Read(f) Save(t)"=FALSE ("Read(f) Write(t)"), "Target Folder Folder"=w244, "Any Config"=w240) -> ("Any Config Out"=w241:T1)  [unwired: 4 in, 4 out]
          n131 = Not Equal?(x=w240, y=w241) -> (x != y?=w239:bool)
          n132 = Bundle By Name(cluster=w245, "Drive Change"=w239, "Config Drive"=w241, "Update Display"=TRUE) -> (w246:T36)
        }
        frame "Config HW Specific Set" {
          n133 = Unbundle By Name(w251) -> ("Config Specific.Specific Data"=w249:T10[], "HW Out.Swerve Read"=w250:T27)
          n134 = Cluster To Array(cluster=w250) -> (array=w247:T16[])
          n135 = for {
            tunnel: w249 -> [w256] mode=indexing
            tunnel: [w257] -> w248 mode=indexing
            tunnel: w247 -> [w255] mode=indexing
            n136 = Unbundle By Name(w255) -> ("Angle"=w254:T18)
            n137 = Bundle By Name(cluster=w256, "Encoder Start Value"=w254) -> (w257:T10)
          }
          n138 = Bundle By Name(cluster=w251, "Config Specific.Specific Data"=w248, "Specific Change"=TRUE) -> (w253:T36)
        }
        frame "Config HW Specific Get" {
          n139 = Unbundle By Name(w262) -> ("Config Specific.Specific Data"=w260:T10[], "HW Out.Swerve Read"=w261:T27)
          n140 = Cluster To Array(cluster=w261) -> (array=w258:T16[])
          n141 = for {
            tunnel: w260 -> [w267] mode=indexing
            tunnel: [w268] -> w259 mode=indexing
            tunnel: w258 -> [w266] mode=indexing
            n142 = Unbundle By Name(w266) -> ("Angle"=w265:T18)
            n143 = Bundle By Name(cluster=w267, "Encoder Start Value"=w265) -> (w268:T10)
          }
          n144 = Bundle By Name(cluster=w262, "Config Specific.Specific Data"=w259, "Specific Change"=TRUE) -> (w264:T36)
        }
        frame "Config HW Specific Save" {
          n145 = Unbundle By Name(w274) -> ("Team Folder"=w273:path, "Config Specific"=w270:T9)
          n146 = call "RWA_File Config.vim"("Read(f) Save(t)"=TRUE ("Read(f) Write(t)"), "Target Folder Folder"=w273, "Any Config"=w270) -> ("Any Config Out"=w269:T9)  [unwired: 4 in, 4 out]
          n147 = Bundle By Name(cluster=w274, "Config Specific"=w269, "Specific Change"=FALSE) -> (w275:T36)
        }
        frame "Config HW Specific Read" {
          n148 = Unbundle By Name(w281) -> ("Team Folder"=w278:path, "Config System"=w280:T20)
          n149 = call "RWA_File Config.vim"("Read(f) Save(t)"=FALSE ("Read(f) Write(t)"), "Target Folder Folder"=w278, "Any Config"=w280) -> ("Any Config Out"=w279:T20)  [unwired: 4 in, 4 out]
          n150 = Bundle By Name(cluster=w281, "Config System"=w279, "Update Display"=TRUE) -> (w282:T36)
        }
        frame "Config System Save" {
          n151 = Unbundle By Name(w288) -> ("Team Folder"=w285:path, "Config System"=w287:T20)
          n152 = call "RWA_File Config.vim"("Read(f) Save(t)"=TRUE ("Read(f) Write(t)"), "Target Folder Folder"=w285, "Any Config"=w287) -> ("Any Config Out"=w286:T20)  [unwired: 4 in, 4 out]
          n153 = Bundle By Name(cluster=w288, "Config System"=w286, "System Change"=FALSE) -> (w289:T36)
        }
        frame "Config System Read" {
          n154 = Unbundle By Name(w295) -> ("Team Folder"=w292:path, "Config System"=w294:T20)
          n155 = call "RWA_File Config.vim"("Read(f) Save(t)"=FALSE ("Read(f) Write(t)"), "Target Folder Folder"=w292, "Any Config"=w294) -> ("Any Config Out"=w293:T20)  [unwired: 4 in, 4 out]
          n156 = Bundle By Name(cluster=w295, "Config System"=w293, "Update Display"=TRUE) -> (w296:T36)
        }
        frame "Config From FP" {
          n157 = Unbundle By Name(w308) -> ("Current Time"=w325:timestamp)
          n158 = Unbundle By Name(w308) -> ("Config Drive"=w314:T1, "Config Drive.Drive HW Ver"=w312:u64, "Config Steer"=w313:T8, "Config Steer.Steer HW Ver"=w310:u64)
          n159 = Unbundle By Name(w308) -> ("Config Specific"=w319:T9, "Config Specific.Specific HW Ver"=w318:u64)
          n160 = Unbundle By Name(w308) -> ("Config System"=w320:T20, "Config System.System Ver"=w322:u64)
          n161 = call "Date Stamp.vi"("Time"=w325) -> ("U64 Out"=w311:u64)  [unwired: 5 in, 1 out]
          n162 = Not Equal?(x=w320, y="Config System") -> (x != y?=w300:bool)
          n163 = Not Equal?(x="Config Specific", y=w319) -> (x != y?=w297:bool)
          n164 = Select(t=w311, s=w300, f=w322) -> (s? t:f=w321:u64)
          n165 = Select(t=w311, s=w297, f=w318) -> (s? t:f=w316:u64)
          n166 = Not Equal?(x="Config Steer", y=w313) -> (x != y?=w298:bool)
          n167 = Bundle By Name(cluster="Config System", "System Ver"=w321) -> (w324:T20)
          n168 = Not Equal?(x="Config Drive", y=w314) -> (x != y?=w301:bool)
          n169 = Select(t=w311, s=w298, f=w310) -> (s? t:f=w302:u64)
          n170 = Bundle By Name(cluster="Config Steer", "Steer HW Ver"=w302) -> (w303:T8)
          n171 = Bundle By Name(cluster="Config Specific", "Specific HW Ver"=w316) -> (w315:T9)
          n172 = Select(t=w311, s=w301, f=w312) -> (s? t:f=w306:u64)
          n173 = Bundle By Name(cluster="Config Drive", "Drive HW Ver"=w306) -> (w305:T1)
          n174 = Bundle By Name(cluster=w308, "Config Drive"=w305, "Drive Change"=w301, "Config Steer"=w303, "Steer Change"=w298, "Config System"=w324, "System Change"=w300, "Config Specific"=w315, "Specific Change"=w297, "Update Display"=TRUE) -> (w309:T36)
        }
        frame "Start HW Steer Set" {
        }
        frame "Default HW Steer Set" {
          n175 = in-place {
            w329 = TRUE ("Drive Change")
            n176 = in-place-cluster #5(w328) -> ("Steer Refs"=w331:T29[])  [unwired: 2 out]
            n177 = for {
              tunnel: w331 -> [w333] mode=indexing
              tunnel: [w332] -> w330 mode=indexing
              n178 = call <vilib>:"CTRE_Phoenix_MotorControl_FactoryDefault.vi"("PhoenixMotorControlDevRef"=w333) -> ("PhoenixMotorControlDevRef"=w332:T29)  [unwired: 9 in, 1 out]
            }
            n179 = in-place-cluster #5("Steer Refs"=w330, "Steer Change"=w329, "Specific Change"=w329) -> (w327:T36)
          }
        }
        frame "Defalut HW Drive Set" {
          n180 = in-place {
            n181 = in-place-cluster #6(w335) -> ("Drive Refs"=w338:T29[])  [unwired: 1 out]
            n182 = for {
              tunnel: w338 -> [w340] mode=indexing
              tunnel: [w339] -> w337 mode=indexing
              n183 = call <vilib>:"SPARK Restore Factory Default.vi"("MotorControlDeviceRef"=w340) -> ("MotorControlDeviceRef"=w339:T29)  [unwired: 9 in, 1 out]
            }
            n184 = in-place-cluster #6("Drive Refs"=w337, "Drive Change"=TRUE) -> (w334:T36)
          }
        }
      }
    }
    n185 = Unbundle By Name(w94) -> ("Config System"=w55:T20, "Config Drive"=w56:T1, "Config Steer"=w91:T8, "Update Display"=w92:bool, "Config System"=w74:T20, "Config Specific"=w63:T9)
    n186 = Unbundle By Name(w94) -> ("State"=w90:T35)
    n187 = Unbundle By Name(w94) -> ("Cycle Time(S)"=w96:dbl)
    "Cycle Time (S)" <- w96
    n188 = Unbundle By Name(w94) -> ("ACT Input"=→"CMD":T13, "HW Out"=w88:T26, "System Output"=w79:T25)
    "HW Output" <- w88
    "System Config" <- w79
    n189 = case shown="\"Startup\", \"Configuring\"" w90 {
      frame "Startup", "Configuring" {
        # "#Fix"
      }
      frame Default {
      }
    }
    n190 = case shown="True" w92 {
      tunnel: w91 -> [_ w490]
      tunnel: w74 -> [_ w492]
      tunnel: w63 -> [_ w491]
      tunnel: w56 -> [_ w489]
      tunnel: w55 -> [_ w488]
      frame False {
      }
      frame True {
        n191 = local write "Config System"(w492) -> ()
        n192 = local write "Config Specific"(w491) -> ()
        n193 = local write "Config Steer"(w490) -> ()
        n194 = local write "Config System"(w488) -> ()
        n195 = local write "Config Drive"(w489) -> ()
      }
    }
    n196 = global write "Global_ACT_Data Out.vi" "ACT_Template_System Output"(w79) -> ()
    n197 = global write "Global_ACT_Data Out.vi" "ACT_Template_HW Output"(w88) -> ()
    n198 = global write "Global_ACT_Data Out.vi" "ACT_Template_CycleTime(S)"(w96) -> ()
    n199 = Bundle By Name(cluster=w94, "Update Display"=FALSE) -> (w97:T36)
  }
  n200 = flat-sequence {
    frame #0 {
      (unwired) ENUM_ACT_State."Startup" ("State")
      (unwired) ENUM_ACT_Action."No Action" ("Action")
      # "State LIST"
      # "Action LIST"
    }
  }
  n201 = Unbundle By Name(w29) -> ("Steer Refs"=w26:T29[], "Drive Refs"=w14:T29[])
  n202 = flat-sequence {
    tunnel: w26 -> [w495]
    tunnel: w14 -> [w494]
    frame #0 {
      n203 = for {
        tunnel: w495 -> [w497] mode=indexing
        tunnel: w494 -> [w496] mode=indexing
        n204 = call <vilib>:"WPI_MotorControlDisable.vi"("MotorControlDevRef"=w496) -> ()  [unwired: 9 in, 2 out]
        n205 = call <vilib>:"WPI_MotorControlDisable.vi"("MotorControlDevRef"=w497) -> ()  [unwired: 9 in, 2 out]
      }
      n206 = local write "CMD Override"(T12."Teleop-Auto" ("CMD Override")) -> ()
    }
  }
